vi "Autonomous Independent.vi"() -> ()   [LabVIEW 2017]
doc: "This VI is called when autonomous begins, and will automatically be terminated when autonomous ends. You can carry out timed or sensor driven robot movement independently without needing to return to the caller."
uses:
  <vilib>/Rock Robotics/Network Tables/NT Write Boolean.vi
  Robot Global Data.vi
  <vilib>/Rock Robotics/Network Tables/NT Read Number.vi
  <vilib>/Rock Robotics/WPI/Utilities/WPI_GetSetVariantRefNum.vi
  <vilib>/addons/control/pid/pid.llb/PID (DBL).vi
  <vilib>/Rock Robotics/WPI/RobotDrive/WPI_RobotDriveArcadeDrive_Standard(NoSaturation).vi
  <vilib>/Rock Robotics/Network Tables/NT Read Boolean.vi
  <vilib>/Rock Robotics/Network Tables/NT Write Number.vi
  <vilib>/addons/control/pid/NI_PID_pid.lvlib
panel:
  in  "PID turn angle gains":T1={"proportional gain (Kc)"=0.07, "integral time (Ti, min)"=0.0, "derivative time (Td, min)"=1e-05}
  in  "PID arm gains":T1={"proportional gain (Kc)"=1.1, "integral time (Ti, min)"=0.008, "derivative time (Td, min)"=0.0001}
  in  "PID control on":bool
  in  "Angle A?":bool=TRUE
  in  "angle A 2":dbl=30.0
  in  "angle B 2":dbl=90.0
  out "Waveform Chart arm":cluster{"angle B 2":dbl, "Arm Angle":dbl, dbl}(graph)
  in  "Chart slowing 2":i32(knob)=3 scale=1.0..10.0
  in  "Shooter control":dbl(slide) scale=-1.0..1.0
  in  "Arm control":dbl(slide) scale=-1.0..1.0
  in  "Chart slowing":i32(knob)=1 scale=1.0..10.0
  in  "angle B":dbl=90.0
  in  "angle A":dbl
  in  "Reset Gyro":bool
  out "Waveform Chart":cluster{"f":dbl, dbl}(graph)
  in  "Which angle?":bool=TRUE
  out "Stop Wheel Loop":bool
  # "Be sure to right-click and choose Data Operations>>Make Current Value default if you want to save the array values with the VI"
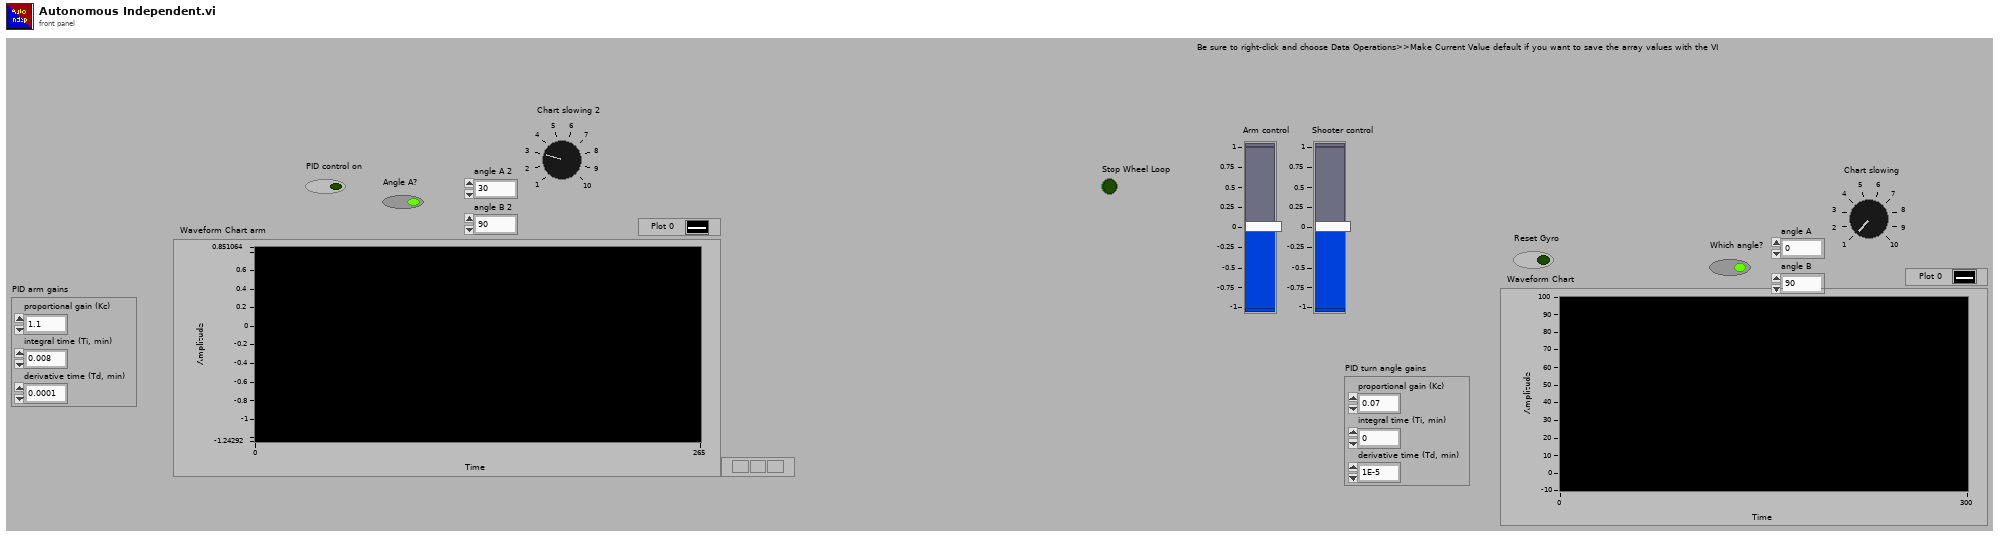
[diagram p1: front panel]
types:
  T1 = cluster{"proportional gain (Kc)":dbl, "integral time (Ti, min)":dbl, "derivative time (Td, min)":dbl}
  T2 = typedef "WPI_GyroDevRef.ctl" = cluster{"DevStatus":errorcluster, "Analog Channel":T3, "Gain (VoltsPerDegree/Second)":dbl, "Gyro Type":enum16{"Analog", "XRS450"}, "Handle":i32, "SPI Bus":T4, "Device Found":bool, "Sample Rate":dbl, "Calibrate On Open":bool, "Offset":dbl}
  T3 = typedef "FPGA_AIChannel.ctl" = enum8{"AI 0", "AI 1", "AI 2", "AI 3", "AI MXP 0", "AI MXP 1", "AI MXP 2", "AI MXP 3", "Invalid"}
  T4 = typedef "spi_bus.ctl" = enum16{"SPI On-Board, CS0", "SPI On-Board, CS1", "SPI On-Board, CS2", "SPI On-Board, CS3", "SPI MXP", "Invalid"}
  T5 = typedef "WPI_PotentiometerDevRef.ctl" = cluster{"DevStatus":errorcluster, "Analog Channel":T3, "Invert Output":bool}
  T6 = typedef "WPI_RobotDriveDevRef.ctl" = cluster{"DevStatus":errorcluster, "Motors[]":T7[], "Square Inputs":bool, "Max Output":dbl}
  T7 = typedef "WPI_MotorControlDeviceRef.ctl" = cluster{"DeviceStatus":errorcluster, "Type":T8, "PWM":cluster{"PWM Channel":T9, "DeadBand":T10}, "CAN":cluster{"Device Number":u8, "SetOutput VI Ref":variant, "GetOutput VI Ref":variant, "Enable VI Ref":variant, "Disable VI Ref":variant, "Data":variant}, "Invert":bool, "DIO PWM":cluster{"PWM \"Enable\" Channel":T9, "DIOChannel":T11, "PWM Rate":dbl}}
  T8 = typedef "WPI_MotorControlType.ctl" = enum16{"PWM", "CAN", "DIO PWM"}
  T9 = typedef "FPGA_DIOPWMChannel.ctl" = enum8{"PWM 0", "PWM 1", "PWM 2", "PWM 3", "PWM 4", "PWM 5", "PWM 6", "PWM 7", "PWM 8", "PWM 9", "PWM MXP 0", "PWM MXP 1", "PWM MXP 2", "PWM MXP 3", "PWM MXP 4", "PWM MXP 5", "PWM MXP 6", "PWM MXP 7", "PWM MXP 8", "PWM MXP 9", "Invalid"}
  T10 = typedef "WPI_PWMDeadband.ctl" = cluster{"Name":string, "maxPositivePwm":i32, "minPositivePwm":i32, "centerPwm":i32, "maxNegativePwm":i32, "minNegativePwm":i32, "angularRange":u16}
  T11 = typedef "FPGA_DIOChannel.ctl" = enum8{"DIO 0", "DIO 1", "DIO 2", "DIO 3", "DIO 4", "DIO 5", "DIO 6", "DIO 7", "DIO 8", "DIO 9", "DIO MXP 0", "DIO MXP 1", "DIO MXP 2", "DIO MXP 3", "DIO MXP 4", "DIO MXP 5", "DIO MXP 6", "DIO MXP 7", "DIO MXP 8", "DIO MXP 9", "DIO MXP 10", "DIO MXP 11", "DIO MXP 12", "DIO MXP 13", "DIO MXP 14", "DIO MXP 15", "SPI Port CS1", "SPI Port CS2", "SPI Port CS3", "SPI Port MISO", "SPI Port MOSI", "Invalid"}
  T12 = typedef "WPI_SwitchDevRef.ctl" = cluster{"DevStatus":errorcluster, "DIO Channel":T11, "CntIndex":T13, "Normally Closed":bool}
  T13 = typedef "FPGA_CounterCtrSystemIndex.ctl" = enum8{"Ctr 0", "Ctr 1", "Ctr 2", "Ctr 3", "Ctr 4", "Ctr 5", "Ctr 6", "Ctr 7", "Invalid"}
  T14 = typedef "WPI_AccelerometerDevRef.ctl" = cluster{"DevStatus":errorcluster, "Scaling":T15, "Analog Channels":T16, "I2C Bus":T17, "SPI Bus":T4, "Accel Range":T18, "ADXL Axes":T19, "Handle":i32, "Device Address":u8, "Accel Type":enum16{"Analog", "ADXL345 I2C", "ADXL345 SPI", "Internal", "ADXL362 SPI"}}
  T15 = typedef "WPI_AccelerometerScaling.ctl" = cluster{"Gain (VoltsPerG)":dbl, "Center Voltage":dbl}
  T16 = typedef "WPI_AccelerometerAnalogChannels.ctl" = cluster{"X-Axis":T3, "Y-Axis":T3, "Z-Axis":T3}
  T17 = typedef "i2c_bus.ctl" = enum16{"I2C On-Board", "I2C MXP", "Invalid"}
  T18 = typedef "ADXL345 Range.ctl" = u8
  T19 = typedef "WPI_AccelerometerADXL345 Axes.ctl" = cluster{"X-Axis":bool, "Y-Axis":bool, "Z-Axis":bool}
  T20 = cluster{"X-Axis":dbl, "Y-Axis":dbl, "Z-Axis":dbl}
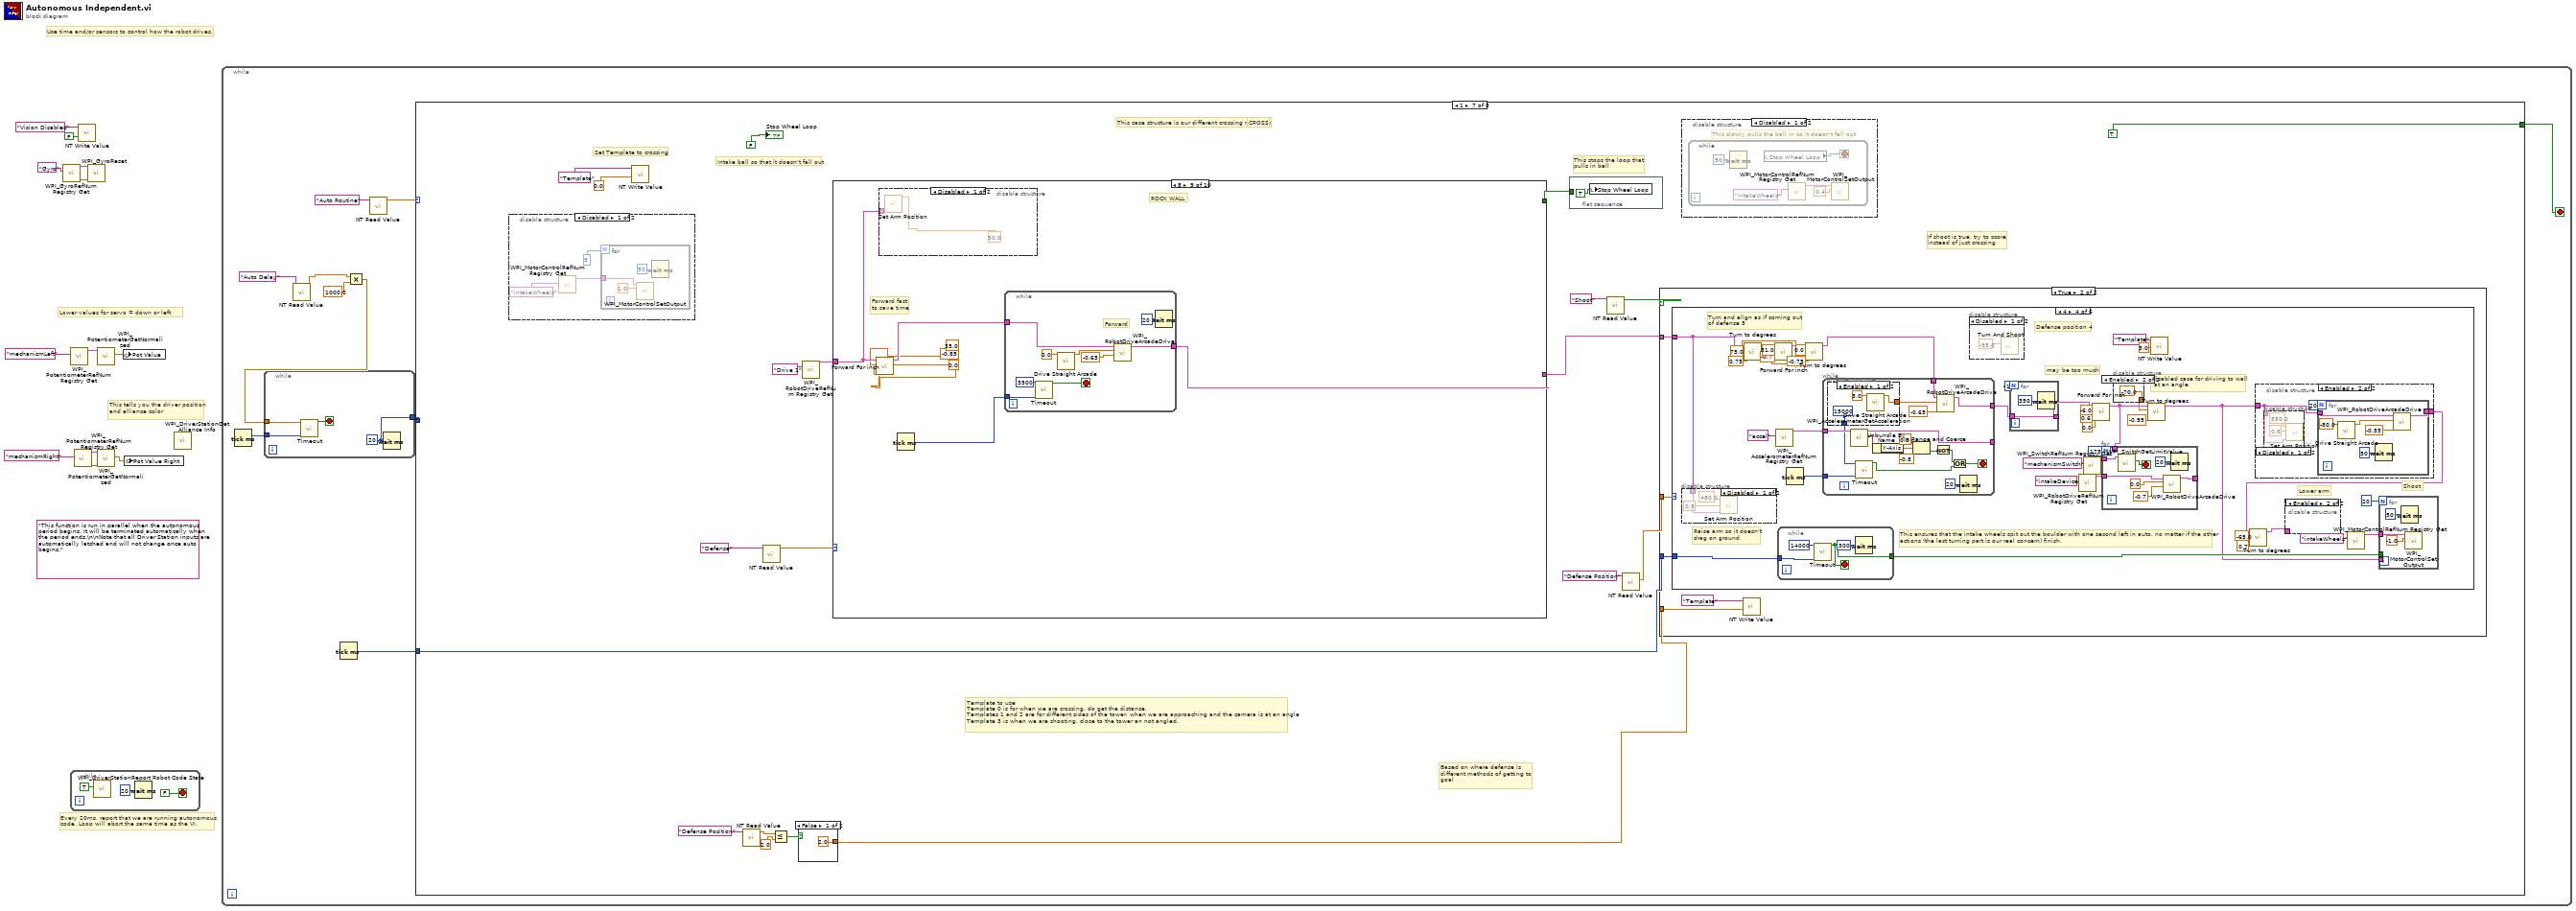
[diagram p0: block diagram]
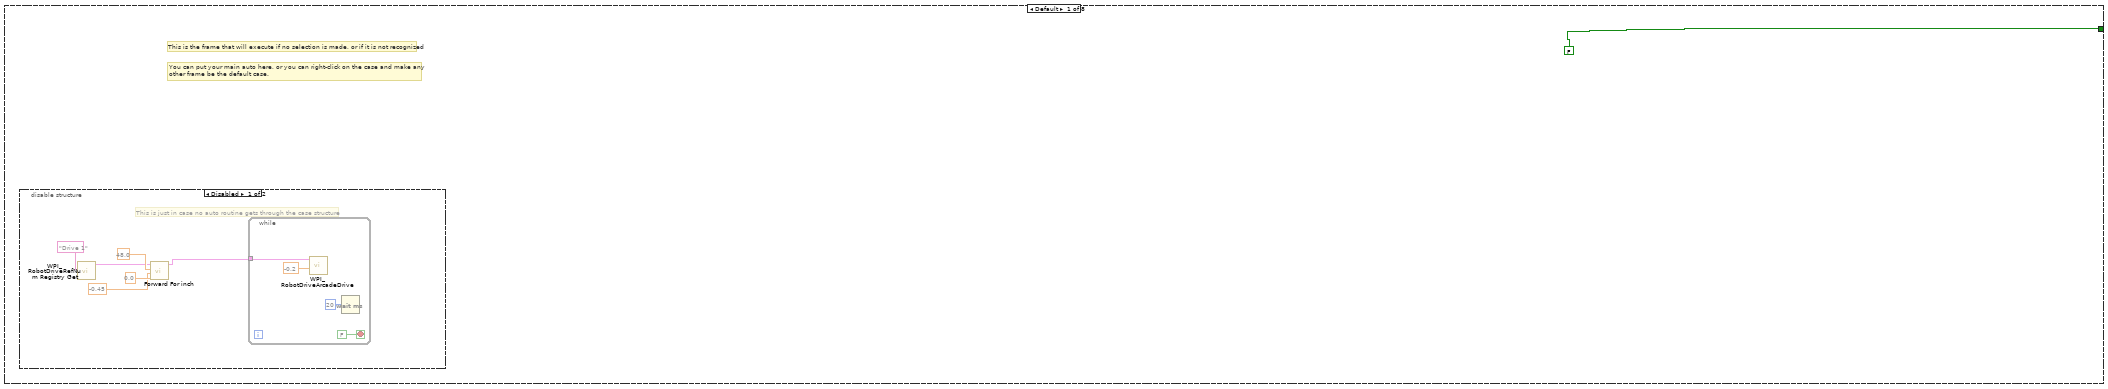
[diagram p2: hidden frame]
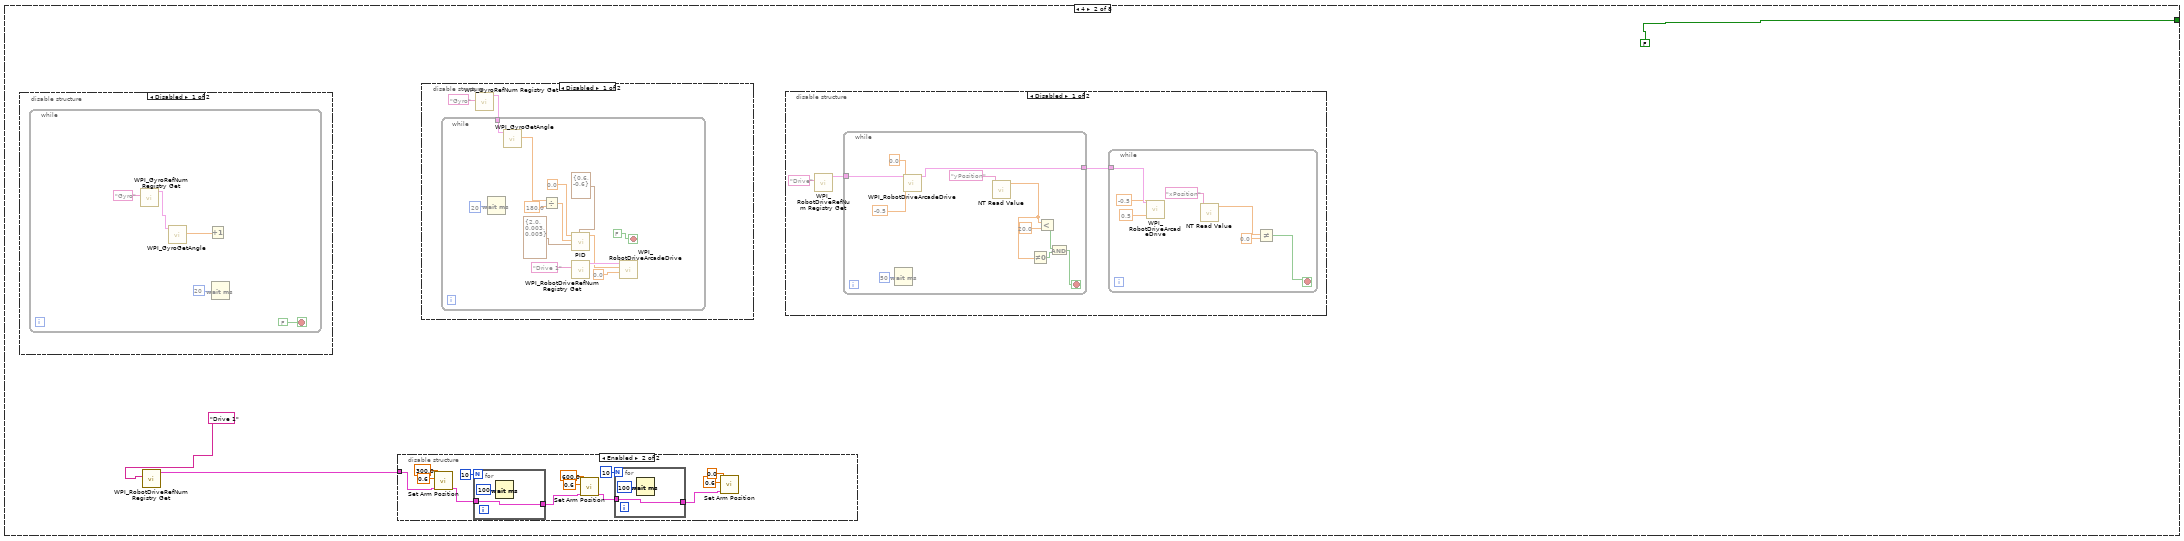
[diagram p4: hidden frame]
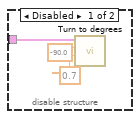
[diagram p5: hidden frame]
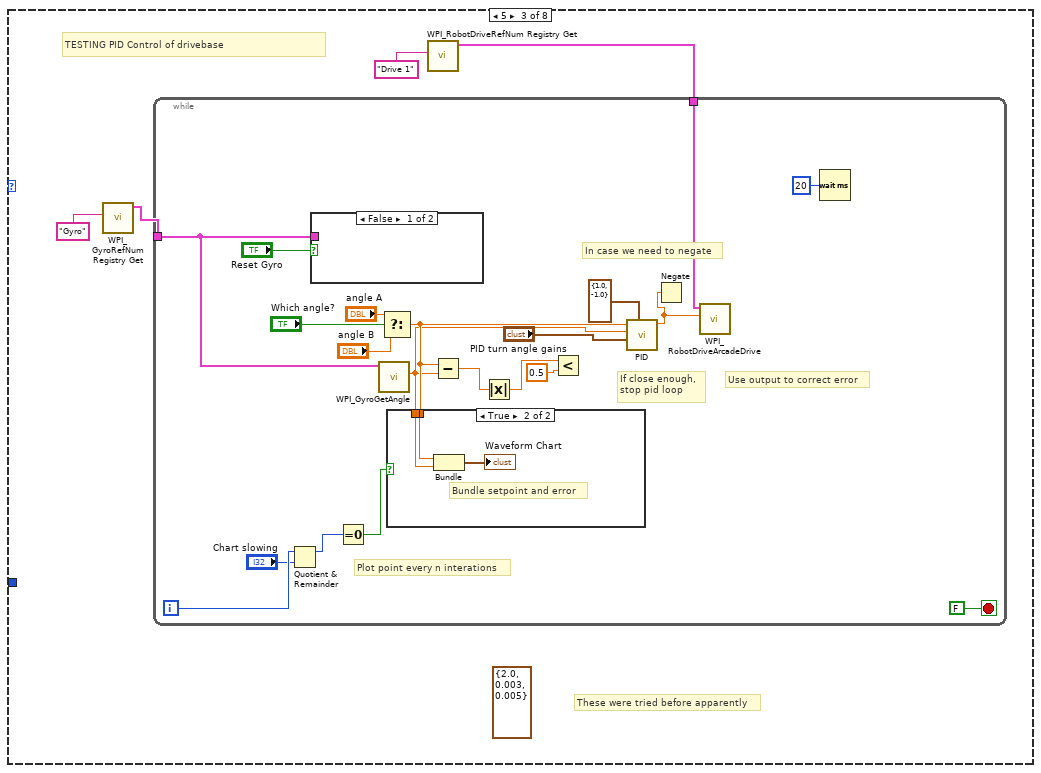
[diagram p9: hidden frame]
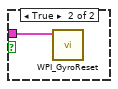
[diagram p11: hidden frame]
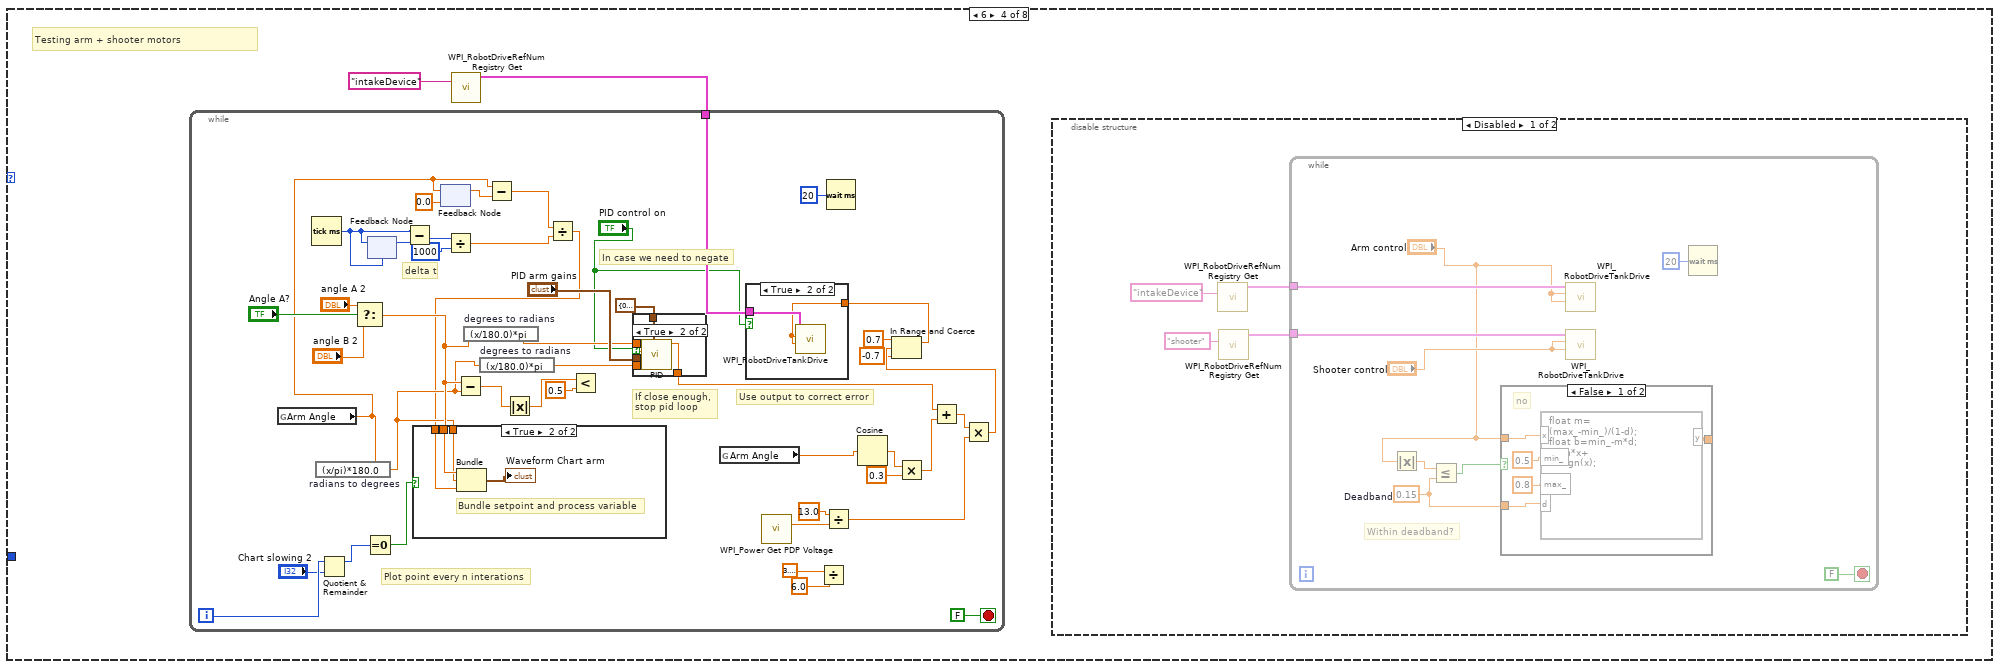
[diagram p12: hidden frame]
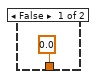
[diagram p14: hidden frame]
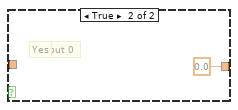
[diagram p16: hidden frame]
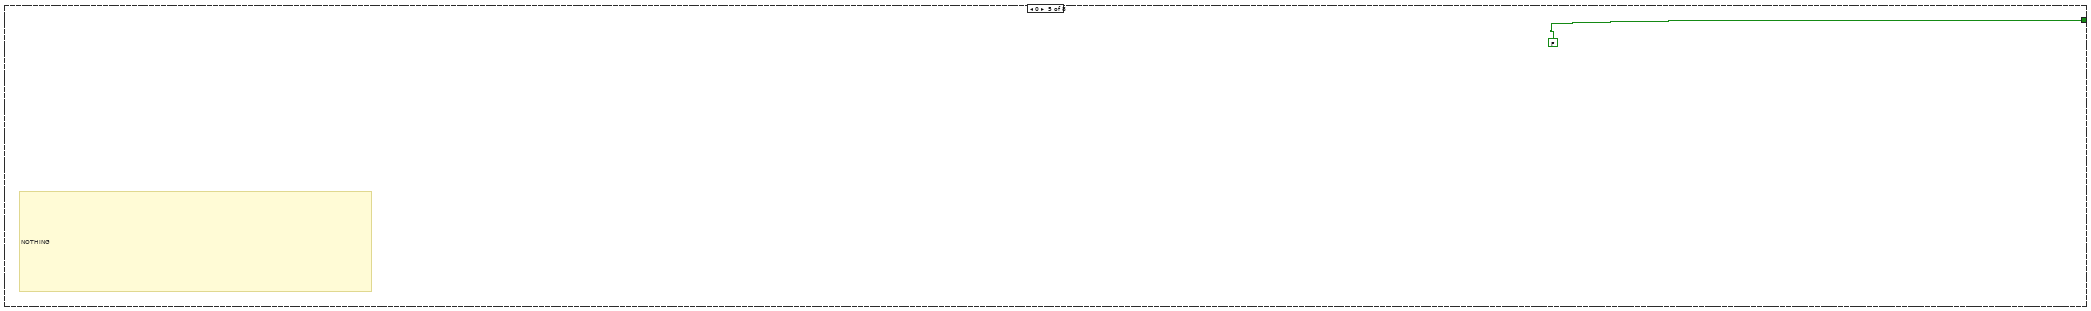
[diagram p18: hidden frame]
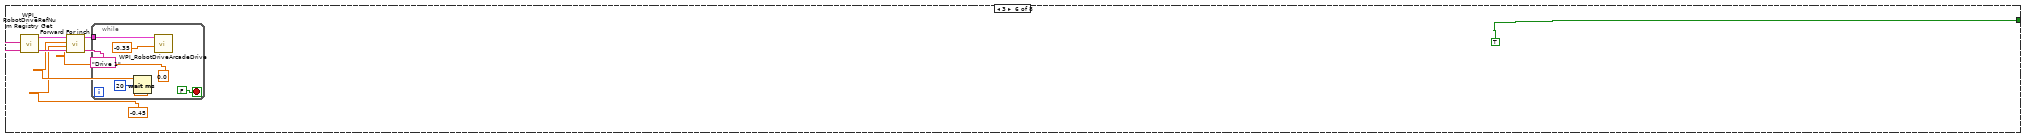
[diagram p19: hidden frame]
diagram:
  (unwired) "This function is run in parallel when the autonomous period begins. It will be terminated automatically when the period ends.\n\nNote that all Driver Station inputs are automatically latched and will not change once auto begins."
  # "Lower values for servo = down or left"
  # "Use time and/or sensors to control how the robot drives."
  # "Every 20ms, report that we are running autonomous\ncode. Loop will abort the same time as the VI."
  # "This tells you the driver position\nand alliance color"
  n1 = call <vilib>:"WPI_GyroRefNum Registry Get.vi"("refnum name"="Gyro") -> ("error out"=w12:errorcluster, "GyroDevRef"=w11:T2)  [unwired: 9 in]
  n2 = while {
    stop <- FALSE stop-if-true
    n3 = call <vilib>:"WPI_DriverStationReport Robot Code State.vi"("Autonomous"=TRUE) -> ()  [unwired: 10 in, 1 out]
    n4 = Wait (ms)(milliseconds to wait=u32 20) -> ()  [unwired: 1 out]
  }
  n5 = call <vilib>:"WPI_PotentiometerRefNum Registry Get.vi"("refnum name"="mechanismLeft") -> ("PotDevRef"=w4:T5)  [unwired: 9 in, 1 out]
  n6 = call <vilib>:"WPI_PotentiometerRefNum Registry Get.vi"("refnum name"="mechanismRight") -> ("error out"=w3:errorcluster, "PotDevRef"=w2:T5)  [unwired: 9 in]
  n7 = call-poly <vilib>:"NT Write Value.vi"("Boolean"=FALSE, "Name"="Vision Disabled") -> ()  [unwired: 9 in, 1 out]
  n8 = call <vilib>:"WPI_GyroReset.vi"("error in"=w12, "GyroDevRef"=w11) -> ()  [unwired: 8 in, 2 out]
  n9 = call <vilib>:"WPI_PotentiometerGetNormalized.vi"("PotDevRef"=w4) -> ("Normalized Value"=w7:dbl)  [unwired: 8 in, 2 out]
  n10 = call <vilib>:"WPI_PotentiometerGetNormalized.vi"("error in"=w3, "PotDevRef"=w2) -> ("Normalized Value"=w1:dbl)  [unwired: 7 in, 2 out]
  n11 = global write "Robot Global Data.vi" "Pot Value"(w7) -> ()
  n12 = global write "Robot Global Data.vi" "Pot Value Right"(w1) -> ()
  n13 = call <vilib>:"WPI_DriverStationGet Alliance Info.vi"() -> ()  [unwired: 12 out]
  n14 = while {
    stop <- w24 stop-if-true
    n15 = Tick Count (ms)() -> (millisecond timer value=w23:u32)
    n16 = call-poly <vilib>:"NT Read Value.vi"("Name"="Auto Delay") -> ("Numeric"=w20:dbl)  [unwired: 9 in, 1 out]
    n17 = Tick Count (ms)() -> (millisecond timer value=w17:u32)
    n18 = Multiply(x=w20, y=1000.0) -> (x*y=w18:dbl)
    n19 = while {
      tunnel: w23 -> [w29]
      tunnel: [w27] -> w22
      tunnel: w18 -> [w26]
      stop <- w28 stop-if-true
      w27 = u32 20 ("milliseconds to wait")
      n20 = call "Timeout.vi"("Start Time In"=w29, "Time Limit"=w26) -> ("Timeout"=w28:bool)  [unwired: 8 in, 1 out]
      n21 = Wait (ms)(milliseconds to wait=w27) -> ()  [unwired: 1 out]
    }
    n22 = call-poly <vilib>:"NT Read Value.vi"("Name"="Auto Routine") -> ("Numeric"=w16:dbl)  [unwired: 9 in, 1 out]
    n23 = case shown="1" w16 {
      tunnel: [FALSE FALSE _ _ FALSE TRUE TRUE TRUE] -> w24
      tunnel: w22 -> [_ _ _ _ _ _ _ _]
      tunnel: w17 -> [_ _ _ _ _ _ w223 _]
      frame Default {
        # "You can put your main auto here, or you can right-click on the case and make any\nother frame be the default case."
        # "This is the frame that will execute if no selection is made, or if it is not recognized"
        n24 = disable-structure shown="Disabled" {
          frame Disabled {
            # "This is just in case no auto routine gets through the case structure"
            n25 = call <vilib>:"WPI_RobotDriveRefNum Registry Get.vi"("refnum name"="Drive 1") -> ("RobotDriveDevRef"=w32:T6)  [unwired: 9 in, 1 out]
            n26 = call "Forward For inch.vi"("Angle robot facing"=0.0, "Speed"=-0.45, "Distance"=48.0, "RobotDriveDevRef in"=w32) -> ("RobotDriveDevRef out"=w36:T6)  [unwired: 7 in]
            n27 = while {
              tunnel: w36 -> [w38]
              stop <- FALSE stop-if-true
              n28 = call-poly <vilib>:"WPI_RobotDriveArcadeDrive.vi"("Y axis value"=-0.2, "RobotDriveDevRef"=w38) -> ()  [unwired: 7 in, 3 out]
              n29 = Wait (ms)(milliseconds to wait=u32 20) -> ()  [unwired: 1 out]
            }
          }
          frame Enabled {
          }
        }
      }
      frame 4 {
        n30 = disable-structure shown="Disabled" {
          frame Disabled {
            n31 = while {
              stop <- FALSE stop-if-true
              n32 = call <vilib>:"WPI_GyroRefNum Registry Get.vi"("refnum name"="Gyro") -> ("GyroDevRef"=w65:T2)  [unwired: 9 in, 1 out]
              n33 = call <vilib>:"WPI_GyroGetAngle.vi"("GyroDevRef"=w65) -> ("Angle"=w66:dbl)  [unwired: 6 in, 4 out]
              n34 = Increment(x=w66) -> ()  [unwired: 1 out]
              n35 = Wait (ms)(milliseconds to wait=u32 20) -> ()  [unwired: 1 out]
            }
          }
          frame Enabled {
          }
        }
        n36 = call <vilib>:"WPI_RobotDriveRefNum Registry Get.vi"("refnum name"="Drive 1") -> ("RobotDriveDevRef"=w41:T6)  [unwired: 9 in, 1 out]
        n37 = disable-structure shown="Enabled" {
          disable-tunnel: w41 -> [w44 w59]
          frame Disabled {
            n38 = call "Turn to degrees.vi"("Speed/Direction"=0.7, "Angle"=-90.0, "RobotDriveDevRef in"=w44) -> ()  [unwired: 8 in, 1 out]
          }
          frame Enabled {
            n39 = call "Set Arm Position.vi"("RobotDriveDevRef 2"=w59, "Speed"=0.6, "Setpoint"=300.0) -> ("RobotDriveDevRef"=w52:T6)  [unwired: 8 in]
            n40 = for {
              N: 10 -> [_]
              tunnel: [w62] -> w53
              tunnel: w52 -> [w62]
              n41 = Wait (ms)(milliseconds to wait=u32 100) -> ()  [unwired: 1 out]
            }
            n42 = call "Set Arm Position.vi"("RobotDriveDevRef 2"=w53, "Speed"=0.6, "Setpoint"=600.0) -> ("RobotDriveDevRef"=w47:T6)  [unwired: 8 in]
            n43 = for {
              N: 10 -> [_]
              tunnel: [w60] -> w48
              tunnel: w47 -> [w60]
              n44 = Wait (ms)(milliseconds to wait=u32 100) -> ()  [unwired: 1 out]
            }
            n45 = call "Set Arm Position.vi"("RobotDriveDevRef 2"=w48, "Speed"=0.6, "Setpoint"=0.0) -> ()  [unwired: 8 in, 1 out]
          }
        }
        n46 = disable-structure shown="Disabled" {
          frame Disabled {
            n47 = call <vilib>:"WPI_GyroRefNum Registry Get.vi"("refnum name"="Gyro") -> ("GyroDevRef"=w90:T2)  [unwired: 9 in, 1 out]
            n48 = while {
              tunnel: w90 -> [w101]
              stop <- FALSE stop-if-true
              n49 = Wait (ms)(milliseconds to wait=u32 20) -> ()  [unwired: 1 out]
              n50 = call <vilib>:"WPI_GyroGetAngle.vi"("GyroDevRef"=w101) -> ("Angle"=w103:dbl)  [unwired: 6 in, 4 out]
              n51 = Divide(x=w103, y=180.0) -> (x/y=w93:dbl)
              n52 = call-poly <vilib>:"PID.vi"("output range"=cluster{"output high":dbl, "output low":dbl} {"output high"=0.6, "output low"=-0.6}, "PID gains"=T1 {"proportional gain (Kc)"=2.0, "integral time (Ti, min)"=0.003, "derivative time (Td, min)"=0.005} ("Drive straight"), "process variable"=w93, "setpoint"=0.0) -> ("output"=w92:dbl)  [unwired: 6 in, 1 out]
              n53 = call <vilib>:"WPI_RobotDriveRefNum Registry Get.vi"("refnum name"="Drive 1") -> ("RobotDriveDevRef"=w99:T6)  [unwired: 1 in, 9 out]
              n54 = call-poly <vilib>:"WPI_RobotDriveArcadeDrive.vi"("Y axis value"=0.0, "X axis value"=w92, "RobotDriveDevRef"=w99) -> ()  [unwired: 6 in, 3 out]
            }
          }
          frame Enabled {
          }
        }
        n55 = disable-structure shown="Disabled" {
          frame Disabled {
            n56 = call <vilib>:"WPI_RobotDriveRefNum Registry Get.vi"("refnum name"="Drive") -> ("RobotDriveDevRef"=w70:T6)  [unwired: 9 in, 1 out]
            n57 = while {
              tunnel: w70 -> [w86]
              tunnel: [w84] -> w69
              stop <- w79 stop-if-true
              n58 = Wait (ms)(milliseconds to wait=u32 50) -> ()  [unwired: 1 out]
              n59 = call-poly <vilib>:"WPI_RobotDriveArcadeDrive.vi"("Y axis value"=-0.5, "X axis value"=0.0, "RobotDriveDevRef"=w86) -> ("RobotDriveDevRef"=w84:T6)  [unwired: 6 in, 2 out]
              n60 = call-poly <vilib>:"NT Read Value.vi"("Name"="yPosition") -> ("Numeric"=w81:dbl)  [unwired: 9 in, 1 out]
              n61 = Not Equal To 0?(x=w81) -> (x != 0?=w80:bool)
              n62 = Less?(x=w81, y=20.0) -> (x < y?=w82:bool)
              n63 = And(x=w82, y=w80) -> (x .and. y?=w79:bool)
            }
            n64 = while {
              tunnel: w69 -> [w78]
              stop <- w74 stop-if-true
              n65 = call-poly <vilib>:"WPI_RobotDriveArcadeDrive.vi"("Y axis value"=0.5, "X axis value"=-0.5, "RobotDriveDevRef"=w78) -> ()  [unwired: 6 in, 3 out]
              n66 = call-poly <vilib>:"NT Read Value.vi"("Name"="xPosition") -> ("Numeric"=w76:dbl)  [unwired: 9 in, 1 out]
              n67 = Not Equal?(x=w76, y=0.0) -> (x != y?=w74:bool)
            }
          }
          frame Enabled {
          }
        }
      }
      frame 5 {
        (unwired) T1 {"proportional gain (Kc)"=2.0, "integral time (Ti, min)"=0.003, "derivative time (Td, min)"=0.005} ("Drive straight")
        # "These were tried before apparently"
        # "TESTING PID Control of drivebase"
        n68 = call <vilib>:"WPI_GyroRefNum Registry Get.vi"("refnum name"="Gyro") -> ("GyroDevRef"=w108:T2)  [unwired: 9 in, 1 out]
        n69 = call <vilib>:"WPI_RobotDriveRefNum Registry Get.vi"("refnum name"="Drive 1") -> ("RobotDriveDevRef"=w105:T6)  [unwired: 9 in, 1 out]
        n70 = while {
          tunnel: w108 -> [w112]
          tunnel: w105 -> [w111]
          i -> [w114]
          stop <- FALSE stop-if-true
          # "In case we need to negate"
          # "Plot point every n interations"
          # "If close enough,\nstop pid loop"
          # "Use output to correct error"
          n71 = Quotient & Remainder(x=w114, y="Chart slowing") -> (x-y*floor(x/y)=w116:i32)  [unwired: 1 out]
          n72 = case shown="False" "Reset Gyro" {
            tunnel: w112 -> [_ w132]
            frame False {
            }
            frame True {
              n73 = call <vilib>:"WPI_GyroReset.vi"("GyroDevRef"=w132) -> ()  [unwired: 9 in, 2 out]
            }
          }
          n74 = Equal To 0?(x=w116) -> (x = 0?=w115:bool)
          n75 = call <vilib>:"WPI_GyroGetAngle.vi"("GyroDevRef"=w112) -> ("Angle"=w124:dbl)  [unwired: 6 in, 4 out]
          n76 = Select(t="angle A", s="Which angle?", f="angle B") -> (s? t:f=w126:dbl)
          n77 = case shown="True" w115 {
            tunnel: w126 -> [_ w130]
            tunnel: w124 -> [_ w129]
            frame False {
            }
            frame True {
              # "Bundle setpoint and error"
              n78 = Bundle("angle B"=w130, "Angle"=w129) -> (→"Waveform Chart":cluster{"angle B":dbl, "Angle":dbl})  [unwired: 1 in]
            }
          }
          n79 = Subtract(x=w126, y=w124) -> (x-y=w122:dbl)
          n80 = Absolute Value(x=w122) -> (abs(x)=w121:dbl)
          n81 = Less?(x=w121, y=0.5) -> ()  [unwired: 1 out]
          n82 = call-poly <vilib>:"PID.vi"("output range"=cluster{"output high":dbl, "output low":dbl} {"output high"=1.0, "output low"=-1.0}, "PID gains"="PID turn angle gains", "process variable"=w124, "setpoint"=w126) -> ("output"=w110:dbl)  [unwired: 6 in, 1 out]
          n83 = Negate(x=w110) -> ()  [unwired: 1 out]
          n84 = call-poly <vilib>:"WPI_RobotDriveArcadeDrive.vi"("X axis value"=w110, "RobotDriveDevRef"=w111) -> ()  [unwired: 7 in, 3 out]
          n85 = Wait (ms)(milliseconds to wait=u32 20) -> ()  [unwired: 1 out]
        }
      }
      frame 6 {
        # "Testing arm + shooter motors"
        n86 = call <vilib>:"WPI_RobotDriveRefNum Registry Get.vi"("refnum name"="intakeDevice") -> ("RobotDriveDevRef"=w134:T6)  [unwired: 9 in, 1 out]
        n87 = while {
          tunnel: w134 -> [w166]
          i -> [w168]
          stop <- FALSE stop-if-true
          # "delta t"
          # "In case we need to negate"
          # "Plot point every n interations"
          # "If close enough,\nstop pid loop"
          # "Use output to correct error"
          n88 = global read "Robot Global Data.vi" "Arm Angle"() -> (w136:dbl)
          n89 = Tick Count (ms)() -> (millisecond timer value=w143:u32)
          n90 = expression code="(x/pi)*180.0" "radians to degrees"(w136) -> (w145:dbl)
          n91 = Quotient & Remainder(x=w168, y="Chart slowing 2") -> (x-y*floor(x/y)=w170:i32)  [unwired: 1 out]
          n92 = Select(t="angle A 2", s="Angle A?", f="angle B 2") -> (s? t:f=w160:dbl)
          n93 = Equal To 0?(x=w170) -> (x = 0?=w169:bool)
          n94 = feedback #1(w143) -> (w144:u32)
          n95 = feedback-in #1(w143) -> ()
          n96 = Subtract(x=w143, y=w144) -> (x-y=w142:u32)
          n97 = feedback #2(0.0 ("Arm Angle")) -> (w140:dbl)
          n98 = feedback-in #2(w136) -> ()
          n99 = Divide(x=w142, y=u32 1000) -> (x/y=w137:dbl)
          n100 = Subtract(x=w160, y=w145) -> (x-y=w159:dbl)
          n101 = expression code="(x/180.0)*pi" "degrees to radians"(w160) -> (w161:dbl)
          n102 = expression code="(x/180.0)*pi" "degrees to radians"(w145) -> (w148:dbl)
          n103 = Subtract(x=w136, y=w140) -> (x-y=w138:dbl)
          n104 = Absolute Value(x=w159) -> (abs(x)=w175:dbl)
          n105 = Divide(x=w138, y=w137) -> (x/y=w135:dbl)
          n106 = case shown="True" w169 {
            tunnel: w160 -> [_ w191]
            tunnel: w145 -> [_ w190]
            tunnel: w135 -> [_ w188]
            frame False {
            }
            frame True {
              # "Bundle setpoint and process variable"
              n107 = Bundle("angle B 2"=w191, "Arm Angle"=w190, w188) -> (→"Waveform Chart arm":cluster{"angle B 2":dbl, "Arm Angle":dbl, dbl})  [unwired: 1 in]
            }
          }
          n108 = Less?(x=w175, y=0.5) -> ()  [unwired: 1 out]
          n109 = case shown="True" "PID control on" {
            tunnel: "PID arm gains" -> [_ w187]
            tunnel: cluster{"output high":dbl, "output low":dbl} {"output high"=0.7, "output low"=-0.7} ("output range") -> [_ w186]
            tunnel: w161 -> [_ w185]
            tunnel: w148 -> [_ w184]
            tunnel: [0.0 ("output") w183] -> w147
            frame False {
            }
            frame True {
              n110 = call-poly <vilib>:"PID.vi"("output range"=w186, "PID gains"=w187, "process variable"=w184, "setpoint"=w185) -> ("output"=w183:dbl)  [unwired: 6 in, 1 out]
            }
          }
          n111 = global read "Robot Global Data.vi" "Arm Angle"() -> (w155:dbl)
          n112 = call <vilib>:"WPI_Power Get PDP Voltage.vi"() -> ("voltage (V)"=w165:dbl)  [unwired: 14 in, 1 out]
          n113 = Divide(x=3.141592653589793, y=6.0) -> ()  [unwired: 1 out]
          n114 = Divide(x=13.0, y=w165) -> (x/y=w153:dbl)
          n115 = Wait (ms)(milliseconds to wait=u32 20) -> ()  [unwired: 1 out]
          n116 = Cosine(x=w155) -> (cos(x)=w158:dbl)
          n117 = Multiply(x=w158, y=0.3) -> (x*y=w156:dbl)
          n118 = Add(x=w147, y=w156) -> (x+y=w154:dbl)
          n119 = Multiply(x=w154, y=w153) -> (x*y=w152:dbl)
          n120 = In Range and Coerce(upper limit=0.7, x=w152, lower limit=-0.7) -> (coerced(x)=w149:dbl)  [unwired: 1 out]
          n121 = case shown="True" "PID control on" {
            tunnel: w166 -> [_ w181]
            tunnel: w149 -> [_ w180]
            frame False {
            }
            frame True {
              n122 = call <vilib>:"WPI_RobotDriveTankDrive.vi"("Right axis value"=w180, "Left axis value"=w180, "RobotDriveDevRef"=w181) -> ()  [unwired: 6 in, 3 out]
            }
          }
        }
        n123 = disable-structure shown="Disabled" {
          frame Disabled {
            n124 = call <vilib>:"WPI_RobotDriveRefNum Registry Get.vi"("refnum name"="intakeDevice") -> ("RobotDriveDevRef"=w195:T6)  [unwired: 9 in, 1 out]
            n125 = call <vilib>:"WPI_RobotDriveRefNum Registry Get.vi"("refnum name"="shooter") -> ("RobotDriveDevRef"=w194:T6)  [unwired: 9 in, 1 out]
            n126 = while {
              tunnel: w195 -> [w203]
              tunnel: w194 -> [w202]
              stop <- FALSE stop-if-true
              w198 = 0.15  # Deadband
              # "Within deadband?"
              n127 = Absolute Value(x="Arm control") -> (abs(x)=w200:dbl)
              n128 = Less Or Equal?(x=w200, y=w198) -> (x <= y?=w199:bool)
              n129 = case shown="False" w199 {
                tunnel: [w209 0.0 ("y")] -> _
                tunnel: "Arm control" -> [w206 _]
                tunnel: w198 -> [w205 _]
                frame False {
                  # "no"
                  n130 = formula code="float m= \n(max_-min_)/(1-d);\nfloat b=min_-m*d;\ny=m*x+\nb*sign(x);"("x"=w206, "min_"=0.5 ("input variable"), "max_"=0.8 ("input variable"), "d"=w205) -> ("y"=w209:dbl)
                }
                frame True {
                  # "Yes"
                  # "Output 0"
                }
              }
              n131 = call <vilib>:"WPI_RobotDriveTankDrive.vi"("Right axis value"="Arm control", "Left axis value"="Arm control", "RobotDriveDevRef"=w203) -> ()  [unwired: 6 in, 3 out]
              n132 = call <vilib>:"WPI_RobotDriveTankDrive.vi"("Right axis value"="Shooter control", "Left axis value"="Shooter control", "RobotDriveDevRef"=w202) -> ()  [unwired: 6 in, 3 out]
              n133 = Wait (ms)(milliseconds to wait=u32 20) -> ()  [unwired: 1 out]
            }
          }
          frame Enabled {
          }
        }
      }
      frame 0 {
        # "NOTHING"
      }
      frame 3 {
        n134 = call <vilib>:"WPI_RobotDriveRefNum Registry Get.vi"("refnum name"="Drive 1") -> ("RobotDriveDevRef"=w217:T6)  [unwired: 9 in, 1 out]
        n135 = call "Forward For inch.vi"("Angle robot facing"=0.0, "Speed"=-0.45, "Distance"=48.0, "RobotDriveDevRef in"=w217) -> ("RobotDriveDevRef out"=w213:T6)  [unwired: 7 in]
        n136 = while {
          tunnel: w213 -> [w220]
          stop <- FALSE stop-if-true
          n137 = Wait (ms)(milliseconds to wait=u32 20) -> ()  [unwired: 1 out]
          n138 = call-poly <vilib>:"WPI_RobotDriveArcadeDrive.vi"("Y axis value"=-0.35, "RobotDriveDevRef"=w220) -> ()  [unwired: 7 in, 3 out]
        }
      }
      frame 1 {
        # "CROSS"
        # "This stops the loop that\npulls in ball"
        # "Based on where defense is\ndifferent methods of getting to\ngoal"
        # "If shoot is true, try to score\ninstead of just crossing"
        # "This case structure is our different crossing methods"
        # "Intake ball so that it doesn't fall out"
        # "Set Template to crossing"
        # "Template to use\nTemplate 0 is for when we are crossing, do get the distance.\nTemplates 1 and 2 are for different sides of the tower, when we are approaching and the camera is at an angle\nTemplate 3 is when we are shooting, close to the tower an not angled."
        n139 = disable-structure shown="Disabled" {
          frame Disabled {
            n140 = call <vilib>:"WPI_MotorControlRefNum Registry Get.vi"("refnum name"="intakeWheels") -> ("MotorControlDevRef"=w248:T7)  [unwired: 9 in, 1 out]
            n141 = for {
              N: 5 -> [_]
              tunnel: w248 -> [w251]
              n142 = call <vilib>:"WPI_MotorControlSetOutput.vi"("Output"=1.0, "MotorControlDevRef"=w251) -> ()  [unwired: 7 in, 3 out]
              n143 = Wait (ms)(milliseconds to wait=u32 50) -> ()  [unwired: 1 out]
            }
          }
          frame Enabled {
          }
        }
        n144 = call-poly <vilib>:"NT Write Value.vi"("Numeric"=0.0, "Name"="Template") -> ()  [unwired: 9 in, 1 out]
        n145 = call-poly <vilib>:"NT Read Value.vi"("Name"="Defense Position") -> ("Numeric"=w229:dbl)  [unwired: 9 in, 1 out]
        n146 = call-poly <vilib>:"NT Read Value.vi"("Name"="Defense") -> ("Numeric"=w240:dbl)  [unwired: 9 in, 1 out]
        n147 = Less Or Equal?(x=w229, y=2.0) -> (x <= y?=w231:bool)
        n148 = case shown="False" w231 {
          tunnel: [2.0 ("Speed/Direction") 1.0 ("Speed/Direction")] -> w227
          frame False {
          }
          frame True {
          }
        }
        n149 = call <vilib>:"WPI_RobotDriveRefNum Registry Get.vi"("refnum name"="Drive 1") -> ("RobotDriveDevRef"=w238:T6)  [unwired: 9 in, 1 out]
        n150 = case shown="8" w240 {
          tunnel: [w257 w264 w290 w413 w500 w514 w528 w537 w554 w566] -> w232
          tunnel: w238 -> [w257 w269 w289 w414 w496 w513 w527 w538 w553 w568]
          tunnel: [FALSE _ _ _ _ _ _ _ _ _] -> w234
          frame 0, Default {
          }
          frame 1 {
            # "If we decide to drive to castle wall at an angle,\nthe code in the enabled structure will be disabled\nand code will be enabled in the next case structure\nit drive at an angle"
            # "Lower arm"
            # "Go under bar, up to align with low goal"
            # "Go forward fast (to save time)"
            # "Pause"
            # "LOW BAR"
            n151 = call <vilib>:"WPI_SwitchRefNum Registry Get.vi"("refnum name"="mechanismSwitch") -> ("SwitchDevRef"=w260:T12)  [unwired: 9 in, 1 out]
            n152 = call <vilib>:"WPI_RobotDriveRefNum Registry Get.vi"("refnum name"="intakeDevice") -> ("RobotDriveDevRef"=w259:T6)  [unwired: 9 in, 1 out]
            n153 = for {
              N: 1 -> [_]
              tunnel: [w287] -> w265
              tunnel: w269 -> [w287]
              n154 = Wait (ms)(milliseconds to wait=u32 350) -> ()  [unwired: 1 out]
            }
            n155 = disable-structure shown="Enabled" {
              disable-tunnel: w269 -> [w279 _]
              disable-tunnel: w260 -> [_ w281]
              disable-tunnel: w259 -> [_ w280]
              frame Disabled {
                n156 = call "Set Arm Position.vi"("RobotDriveDevRef 2"=w279, "Speed"=0.95, "Setpoint"=510.0) -> ()  [unwired: 8 in, 1 out]
              }
              frame Enabled {
                n157 = while {
                  tunnel: w281 -> [w283]
                  tunnel: w280 -> [w282]
                  stop <- w284 stop-if-true
                  n158 = call <vilib>:"WPI_SwitchGetLimitValue.vi"("SwitchDevRef"=w283) -> ("Switch Pressed"=w284:bool)  [unwired: 8 in, 2 out]
                  n159 = call-poly <vilib>:"WPI_RobotDriveArcadeDrive.vi"("Y axis value"=-0.7, "X axis value"=0.0, "RobotDriveDevRef"=w282) -> ()  [unwired: 6 in, 3 out]
                }
              }
            }
            n160 = call "Forward For inch.vi"("Angle robot facing"=0.0, "Speed"=0.78, "Distance"=-32.0, "RobotDriveDevRef in"=w265) -> ("RobotDriveDevRef out"=w263:T6)  [unwired: 7 in]
            n161 = disable-structure shown="Enabled" {
              disable-tunnel: [w272 w276] -> w264
              disable-tunnel: w263 -> [w271 w276]
              frame Enabled {
                n162 = call "Forward For inch.vi"("Angle robot facing"=5.0, "Speed"=0.67, "Distance"=-172.0, "RobotDriveDevRef in"=w271) -> ("RobotDriveDevRef out"=w272:T6)  [unwired: 7 in]
              }
              frame Disabled {
              }
            }
          }
          frame 2 {
            # "PORTCULLIS"
            n163 = disable-structure shown="Enabled" {
              disable-tunnel: [w301 w363] -> w290
              disable-tunnel: w289 -> [w293 w378]
              frame Disabled {
                # "then pause while arm\nlowering"
                # "Pause"
                # "Because we had trouble making it go far\nenough, add a burst of movement at the end"
                # "We think the arm wasn't rasing\nbecause forward for inch wasn't\nending, so we added a time value instead"
                # "I'M SORRY THS IS SO COMPLICATED"
                # "Go forward slowly, so we \ndon't roll off ramp. When arm is high \nenough, start moving forward"
                # "raise arm, and porticullis"
                # "pause"
                # "Go forward to\nporticullus"
                # "Lower arm"
                n164 = for {
                  N: 1 -> [_]
                  tunnel: w293 -> [w358]
                  tunnel: [w358] -> w305
                  n165 = Wait (ms)(milliseconds to wait=u32 750) -> ()  [unwired: 1 out]
                }
                n166 = call "Set Arm Position.vi"("RobotDriveDevRef 2"=w293, "Speed"=0.7, "Setpoint"=700.0) -> ()  [unwired: 8 in, 1 out]
                n167 = global read "Robot Global Data.vi" "Pot Value"() -> (w297:dbl)
                n168 = call <vilib>:"WPI_PotentiometerRefNum Registry Get.vi"("refnum name"="mechanismLeft") -> ("PotDevRef"=w298:T5)  [unwired: 9 in, 1 out]
                n169 = call "Forward For inch.vi"("Angle robot facing"=0.0, "Speed"=-0.5, "Distance"=47.0, "RobotDriveDevRef in"=w305) -> ("RobotDriveDevRef out"=w308:T6)  [unwired: 7 in]
                n170 = call <vilib>:"WPI_RobotDriveRefNum Registry Get.vi"("refnum name"="Drive 1") -> ("RobotDriveDevRef"=w302:T6)  [unwired: 9 in, 1 out]
                n171 = flat-sequence {
                  tunnel: [w313] -> w300
                  tunnel: w294 -> [_]
                  frame #0 {
                    n172 = Tick Count (ms)() -> (millisecond timer value=w313:u32)
                  }
                }
                n173 = for {
                  N: 1 -> [_]
                  tunnel: w308 -> [w360]
                  tunnel: [w360] -> w294
                  n174 = Wait (ms)(milliseconds to wait=u32 200) -> ()  [unwired: 1 out]
                }
                n175 = while {
                  tunnel: w300 -> [w341]
                  tunnel: w294 -> [w336]
                  tunnel: [w335] -> w295
                  stop <- w339 stop-if-true
                  n176 = call "Timeout.vi"("Start Time In"=w341, "Time Limit"=u32 250) -> ("Timeout"=w339:bool)  [unwired: 8 in, 1 out]
                  n177 = call-poly <vilib>:"WPI_RobotDriveArcadeDrive.vi"("Y axis value"=-0.6, "X axis value"=0.0, "RobotDriveDevRef"=w336) -> ("RobotDriveDevRef"=w335:T6)  [unwired: 6 in, 2 out]
                }
                n178 = while {
                  tunnel: w295 -> [w348]
                  tunnel: [w348] -> w296
                  tunnel: w302 -> [w346]
                  tunnel: w298 -> [w345]
                  tunnel: w297 -> [w342]
                  stop <- w349 stop-if-true
                  n179 = call <vilib>:"WPI_PotentiometerGetNormalized.vi"("PotDevRef"=w345) -> ("Normalized Value"=w344:dbl)  [unwired: 8 in, 2 out]
                  n180 = disable-structure shown="Enabled" {
                    disable-tunnel: w344 -> [w352 w355]
                    disable-tunnel: [w351 w353] -> w343
                    disable-tunnel: w342 -> [_ w354]
                    frame Disabled {
                      n181 = expression code="-1505.88*(x-.587)"(w352) -> (w351:dbl)
                    }
                    frame Enabled {
                      n182 = Subtract(x=w355, y=w354) -> (x-y=w357:dbl)
                      n183 = Multiply(x=w357, y=-1505.88) -> (x*y=w353:dbl)
                    }
                  }
                  n184 = Less Or Equal?(x=w343, y=300.0) -> (x <= y?=w349:bool)
                  n185 = call-poly <vilib>:"WPI_RobotDriveArcadeDrive.vi"("Y axis value"=-0.45, "RobotDriveDevRef"=w346) -> ()  [unwired: 7 in, 3 out]
                }
                n186 = call "Set Arm Position.vi"("RobotDriveDevRef 2"=w295, "Speed"=0.8, "Setpoint"=150.0) -> ()  [unwired: 8 in, 1 out]
                n187 = disable-structure shown="Enabled" {
                  disable-tunnel: [w315 w327] -> w301
                  disable-tunnel: w296 -> [w314 w328]
                  frame Disabled {
                    # "Go forward"
                    n188 = Tick Count (ms)() -> (millisecond timer value=w319:u32)
                    n189 = while {
                      tunnel: w319 -> [w326]
                      tunnel: [24.0 ("Distance")] -> w316
                      stop <- w324 stop-if-true
                      n190 = call "Timeout.vi"("Start Time In"=w326, "Time Limit"=u32 10000) -> ("Timeout"=w324:bool)  [unwired: 8 in, 1 out]
                    }
                    n191 = call "Forward For inch.vi"("Angle robot facing"=0.0, "Speed"=-0.7, "Distance"=60.0, "RobotDriveDevRef in"=w314) -> ("RobotDriveDevRef out"=w315:T6)  [unwired: 7 in]
                    n192 = call "Forward For inch.vi"("Angle robot facing"=0.0, "Speed"=-0.65, "Distance"=w316, "RobotDriveDevRef in"=w315) -> ()  [unwired: 7 in, 1 out]
                  }
                  frame Enabled {
                    n193 = for {
                      N: 150 -> [_]
                      tunnel: w328 -> [w332]
                      tunnel: [w330] -> w327
                      n194 = call-poly <vilib>:"WPI_RobotDriveArcadeDrive.vi"("Y axis value"=-0.7, "X axis value"=0.0, "RobotDriveDevRef"=w332) -> ("RobotDriveDevRef"=w330:T6)  [unwired: 6 in, 2 out]
                      n195 = Wait (ms)(milliseconds to wait=u32 20) -> ()  [unwired: 1 out]
                    }
                  }
                }
              }
              frame Enabled {
                # "Go forward"
                # "Wait"
                # "Raise arm"
                # "Forward"
                # "Pause"
                # "Forward"
                # "Lower arm"
                # "Pause"
                n196 = for {
                  N: 1 -> [_]
                  tunnel: w378 -> [w405]
                  tunnel: [w405] -> w374
                  n197 = Wait (ms)(milliseconds to wait=u32 750) -> ()  [unwired: 1 out]
                }
                n198 = call <vilib>:"WPI_SwitchRefNum Registry Get.vi"("refnum name"="mechanismSwitch") -> ("SwitchDevRef"=w382:T12)  [unwired: 9 in, 1 out]
                n199 = call <vilib>:"WPI_RobotDriveRefNum Registry Get.vi"("refnum name"="intakeDevice") -> ("RobotDriveDevRef"=w381:T6)  [unwired: 9 in, 1 out]
                n200 = for {
                  N: 60 -> [_]
                  tunnel: w382 -> [w410]
                  tunnel: w381 -> [w409]
                  tunnel: w378 -> [_]
                  stop <- w408 stop-if-true
                  n201 = call <vilib>:"WPI_SwitchGetLimitValue.vi"("SwitchDevRef"=w410) -> ("Switch Pressed"=w408:bool)  [unwired: 8 in, 2 out]
                  n202 = call-poly <vilib>:"WPI_RobotDriveArcadeDrive.vi"("Y axis value"=-0.7, "X axis value"=0.0, "RobotDriveDevRef"=w409) -> ()  [unwired: 6 in, 3 out]
                  n203 = Wait (ms)(milliseconds to wait=u32 50) -> ()  [unwired: 1 out]
                }
                n204 = call "Forward For inch.vi"("Angle robot facing"=0.0, "Speed"=-0.6, "Distance"=46.0, "RobotDriveDevRef in"=w374) -> ("RobotDriveDevRef out"=w372:T6)  [unwired: 7 in]
                n205 = for {
                  N: 1 -> [_]
                  tunnel: w372 -> [w403]
                  tunnel: [w403] -> w371
                  n206 = Wait (ms)(milliseconds to wait=u32 200) -> ()  [unwired: 1 out]
                }
                n207 = for {
                  N: 6 -> [_]
                  tunnel: w371 -> [w387]
                  tunnel: [w386] -> w366
                  n208 = Wait (ms)(milliseconds to wait=u32 50) -> ()  [unwired: 1 out]
                  n209 = call-poly <vilib>:"WPI_RobotDriveArcadeDrive.vi"("Y axis value"=-0.6, "X axis value"=0.0, "RobotDriveDevRef"=w387) -> ("RobotDriveDevRef"=w386:T6)  [unwired: 6 in, 2 out]
                }
                n210 = call <vilib>:"WPI_RobotDriveRefNum Registry Get.vi"("refnum name"="intakeDevice") -> ("RobotDriveDevRef"=w368:T6)  [unwired: 9 in, 1 out]
                n211 = for {
                  N: 50 -> [_]
                  tunnel: w366 -> [_]
                  tunnel: w368 -> [w399]
                  n212 = call-poly <vilib>:"WPI_RobotDriveArcadeDrive.vi"("Y axis value"=0.8, "X axis value"=0.0, "RobotDriveDevRef"=w399) -> ()  [unwired: 6 in, 3 out]
                  n213 = Wait (ms)(milliseconds to wait=u32 50) -> ()  [unwired: 1 out]
                }
                n214 = for {
                  N: 40 -> [_]
                  tunnel: w366 -> [w395]
                  tunnel: [w395] -> w364
                  n215 = Wait (ms)(milliseconds to wait=u32 20) -> ()  [unwired: 1 out]
                  n216 = call-poly <vilib>:"WPI_RobotDriveArcadeDrive.vi"("Y axis value"=-0.55, "X axis value"=0.0, "RobotDriveDevRef"=w395) -> ()  [unwired: 6 in, 3 out]
                }
                n217 = for {
                  N: 90 -> [_]
                  tunnel: w364 -> [w392]
                  tunnel: [w390] -> w363
                  n218 = call-poly <vilib>:"WPI_RobotDriveArcadeDrive.vi"("Y axis value"=-0.85, "X axis value"=0.0, "RobotDriveDevRef"=w392) -> ("RobotDriveDevRef"=w390:T6)  [unwired: 6 in, 2 out]
                  n219 = Wait (ms)(milliseconds to wait=u32 20) -> ()  [unwired: 1 out]
                }
              }
            }
          }
          frame 3 {
            # "CDF"
            n220 = disable-structure shown="Enabled" {
              disable-tunnel: w414 -> [w429 w459]
              disable-tunnel: [w415 w445] -> w413
              frame Disabled {
                # "Raise arm so it doesn't hit the ground"
                # "Go over"
                # "Very small pause"
                # "While going forward so\nwe don't roll off"
                # "Lower arm onto CDF"
                # "Forward"
                n221 = call "Forward For inch.vi"("Angle robot facing"=0.0, "Speed"=-0.6, "Distance"=38.5, "RobotDriveDevRef in"=w429) -> ("RobotDriveDevRef out"=w420:T6)  [unwired: 7 in]
                n222 = call "Set Arm Position.vi"("RobotDriveDevRef 2"=w420, "Speed"=0.9, "Setpoint"=650.0) -> ("RobotDriveDevRef"=w419:T6)  [unwired: 8 in]
                n223 = for {
                  N: 50 -> [_]
                  tunnel: w420 -> [w432]
                  n224 = Wait (ms)(milliseconds to wait=u32 20) -> ()  [unwired: 1 out]
                  n225 = call-poly <vilib>:"WPI_RobotDriveArcadeDrive.vi"("Y axis value"=-0.35, "X axis value"=0.0 ("Y axis value"), "RobotDriveDevRef"=w432) -> ()  [unwired: 6 in, 3 out]
                }
                n226 = Tick Count (ms)() -> (millisecond timer value=w416:u32)
                n227 = for {
                  N: 5 -> [_]
                  tunnel: [w430] -> w421
                  tunnel: w419 -> [w430]
                  n228 = Wait (ms)(milliseconds to wait=u32 50) -> ()  [unwired: 1 out]
                }
                n229 = while {
                  tunnel: w419 -> [w443]
                  tunnel: [w442] -> w415
                  tunnel: w416 -> [w439]
                  stop <- w438 stop-if-true
                  n230 = call "Timeout.vi"("Start Time In"=w439, "Time Limit"=u32 4000) -> ("Timeout"=w438:bool)  [unwired: 8 in, 1 out]
                  n231 = call "Drive Straight Arcade.vi"("Angle robot facing"=0.0) -> ("Arcade drive x"=w436:dbl)  [unwired: 10 in]
                  n232 = call-poly <vilib>:"WPI_RobotDriveArcadeDrive.vi"("Y axis value"=-0.65, "X axis value"=w436, "RobotDriveDevRef"=w443) -> ("RobotDriveDevRef"=w442:T6)  [unwired: 6 in, 2 out]
                  n233 = Wait (ms)(milliseconds to wait=u32 20) -> ()  [unwired: 1 out]
                }
                n234 = call "Set Arm Position.vi"("RobotDriveDevRef 2"=w421, "Speed"=0.9, "Setpoint"=200.0) -> ()  [unwired: 8 in, 1 out]
              }
              frame Enabled {
                # "forward"
                # "arm up"
                # "While going forward so\nwe don't roll off"
                n235 = call "Forward For inch.vi"("Angle robot facing"=0.0, "Speed"=-0.6, "Distance"=38.0, "RobotDriveDevRef in"=w459) -> ("RobotDriveDevRef out"=w455:T6)  [unwired: 7 in]
                n236 = call <vilib>:"WPI_SwitchRefNum Registry Get.vi"("refnum name"="mechanismSwitch") -> ("SwitchDevRef"=w452:T12)  [unwired: 9 in, 1 out]
                n237 = for {
                  N: 50 -> [_]
                  tunnel: w455 -> [w487]
                  n238 = Wait (ms)(milliseconds to wait=u32 20) -> ()  [unwired: 1 out]
                  n239 = call-poly <vilib>:"WPI_RobotDriveArcadeDrive.vi"("Y axis value"=-0.35, "X axis value"=0.0 ("Y axis value"), "RobotDriveDevRef"=w487) -> ()  [unwired: 6 in, 3 out]
                }
                n240 = call <vilib>:"WPI_RobotDriveRefNum Registry Get.vi"("refnum name"="intakeDevice") -> ("RobotDriveDevRef"=w456:T6)  [unwired: 9 in, 1 out]
                n241 = for {
                  N: 50 -> [_]
                  tunnel: w456 -> [w483]
                  tunnel: w455 -> [w479]
                  tunnel: w452 -> [w481]
                  tunnel: [w480] -> w450
                  tunnel: [w479] -> w446
                  stop <- w482 stop-if-true
                  n242 = call <vilib>:"WPI_SwitchGetLimitValue.vi"("SwitchDevRef"=w481) -> ("Switch Pressed"=w482:bool)  [unwired: 8 in, 2 out]
                  n243 = call-poly <vilib>:"WPI_RobotDriveArcadeDrive.vi"("Y axis value"=-0.8, "X axis value"=0.0, "RobotDriveDevRef"=w483) -> ("RobotDriveDevRef"=w480:T6)  [unwired: 6 in, 2 out]
                  n244 = Wait (ms)(milliseconds to wait=u32 50) -> ()  [unwired: 1 out]
                }
                n245 = Tick Count (ms)() -> (millisecond timer value=w447:u32)
                n246 = while {
                  tunnel: w446 -> [w470]
                  tunnel: [w469] -> w445
                  tunnel: w447 -> [w466]
                  stop <- w465 stop-if-true
                  n247 = call "Timeout.vi"("Start Time In"=w466, "Time Limit"=u32 5000) -> ("Timeout"=w465:bool)  [unwired: 8 in, 1 out]
                  n248 = call "Drive Straight Arcade.vi"("Angle robot facing"=0.0) -> ("Arcade drive x"=w463:dbl)  [unwired: 10 in]
                  n249 = call-poly <vilib>:"WPI_RobotDriveArcadeDrive.vi"("Y axis value"=-0.7, "X axis value"=w463, "RobotDriveDevRef"=w470) -> ("RobotDriveDevRef"=w469:T6)  [unwired: 6 in, 2 out]
                  n250 = Wait (ms)(milliseconds to wait=u32 40) -> ()  [unwired: 1 out]
                }
                n251 = for {
                  N: 5 -> [_]
                  tunnel: [w477] -> w449
                  tunnel: w450 -> [w477]
                  n252 = Wait (ms)(milliseconds to wait=u32 50) -> ()  [unwired: 1 out]
                }
                n253 = for {
                  N: 25 -> [_]
                  tunnel: w449 -> [w473]
                  tunnel: [w472] -> _
                  n254 = call-poly <vilib>:"WPI_RobotDriveArcadeDrive.vi"("Y axis value"=0.7, "X axis value"=0.0, "RobotDriveDevRef"=w473) -> ("RobotDriveDevRef"=w472:T6)  [unwired: 6 in, 2 out]
                  n255 = Wait (ms)(milliseconds to wait=u32 50) -> ()  [unwired: 1 out]
                }
              }
            }
          }
          frame 4 {
            # "Turn to the left, so right wheel hits\nedge of rampart. It is easier to go over\nthis way"
            # "Go forward"
            # "RAMPARTS"
            n256 = disable-structure shown="Disabled" {
              disable-tunnel: w496 -> [w501 _]
              frame Disabled {
                # "Raise arm a little"
                n257 = call "Set Arm Position.vi"("RobotDriveDevRef 2"=w501, "Setpoint"=100.0) -> ()  [unwired: 9 in, 1 out]
              }
              frame Enabled {
              }
            }
            n258 = call "Forward For inch.vi"("Angle robot facing"=0.0, "Speed"=-0.65, "Distance"=30.0, "RobotDriveDevRef in"=w496) -> ("RobotDriveDevRef out"=w495:T6)  [unwired: 7 in]
            n259 = call "Turn to degrees.vi"("Speed/Direction"=0.63, "Angle"=-7.0, "RobotDriveDevRef in"=w495) -> ("RobotDriveDevRef out"=w499:T6)  [unwired: 8 in]
            n260 = Tick Count (ms)() -> (millisecond timer value=w491:u32)
            n261 = while {
              tunnel: [w510] -> w500
              tunnel: w499 -> [w506]
              tunnel: w491 -> [w504]
              stop <- w503 stop-if-true
              # "Forward until over"
              n262 = call "Timeout.vi"("Start Time In"=w504, "Time Limit"=u32 4000) -> ("Timeout"=w503:bool)  [unwired: 8 in, 1 out]
              n263 = call "Drive Straight Arcade.vi"("Angle robot facing"=-5.0) -> ("Arcade drive x"=w508:dbl)  [unwired: 10 in]
              n264 = Wait (ms)(milliseconds to wait=u32 20) -> ()  [unwired: 1 out]
              n265 = call-poly <vilib>:"WPI_RobotDriveArcadeDrive.vi"("Y axis value"=-0.68, "X axis value"=w508, "RobotDriveDevRef"=w506) -> ("RobotDriveDevRef"=w510:T6)  [unwired: 6 in, 2 out]
            }
          }
          frame 5 {
            # "MOAT"
            n266 = Tick Count (ms)() -> (millisecond timer value=w512:u32)
            n267 = disable-structure shown="Disabled" {
              disable-tunnel: w513 -> [w515 _]
              frame Disabled {
                # "Raise arm"
                n268 = call "Set Arm Position.vi"("RobotDriveDevRef 2"=w515, "Setpoint"=50.0) -> ()  [unwired: 9 in, 1 out]
              }
              frame Enabled {
              }
            }
            n269 = while {
              tunnel: w513 -> [w523]
              tunnel: [w524] -> w514
              tunnel: w512 -> [w519]
              stop <- w517 stop-if-true
              # "Go forward"
              n270 = call "Timeout.vi"("Start Time In"=w519, "Time Limit"=u32 5000) -> ("Timeout"=w517:bool)  [unwired: 8 in, 1 out]
              n271 = call "Drive Straight Arcade.vi"("Angle robot facing"=0.0) -> ("Arcade drive x"=w520:dbl)  [unwired: 10 in]
              n272 = call-poly <vilib>:"WPI_RobotDriveArcadeDrive.vi"("Y axis value"=-0.75, "X axis value"=w520, "RobotDriveDevRef"=w523) -> ("RobotDriveDevRef"=w524:T6)  [unwired: 6 in, 2 out]
              n273 = Wait (ms)(milliseconds to wait=u32 20) -> ()  [unwired: 1 out]
            }
          }
          frame 6 {
            # "DRAWBRIDGE"
            n274 = Tick Count (ms)() -> (millisecond timer value=w526:u32)
            n275 = while {
              tunnel: w527 -> [w533]
              tunnel: [w534] -> w528
              tunnel: w526 -> [w530]
              stop <- w529 stop-if-true
              n276 = call "Timeout.vi"("Start Time In"=w530, "Time Limit"=u32 4000) -> ("Timeout"=w529:bool)  [unwired: 8 in, 1 out]
              n277 = call-poly <vilib>:"WPI_RobotDriveArcadeDrive.vi"("Y axis value"=-0.6, "X axis value"=0.0 ("Y axis value"), "RobotDriveDevRef"=w533) -> ("RobotDriveDevRef"=w534:T6)  [unwired: 6 in, 2 out]
              n278 = Wait (ms)(milliseconds to wait=u32 20) -> ()  [unwired: 1 out]
            }
          }
          frame 7 {
            # "SALLY PORT"
            n279 = Tick Count (ms)() -> (millisecond timer value=w539:u32)
            n280 = while {
              tunnel: w538 -> [w544]
              tunnel: [w545] -> w537
              tunnel: w539 -> [w541]
              stop <- w540 stop-if-true
              n281 = call "Timeout.vi"("Start Time In"=w541, "Time Limit"=u32 4000) -> ("Timeout"=w540:bool)  [unwired: 8 in, 1 out]
              n282 = call-poly <vilib>:"WPI_RobotDriveArcadeDrive.vi"("Y axis value"=-0.6, "X axis value"=0.0 ("Y axis value"), "RobotDriveDevRef"=w544) -> ("RobotDriveDevRef"=w545:T6)  [unwired: 6 in, 2 out]
              n283 = Wait (ms)(milliseconds to wait=u32 20) -> ()  [unwired: 1 out]
            }
          }
          frame 8 {
            # "ROCK WALL"
            # "Forward fast\nto save time"
            n284 = call "Forward For inch.vi"("Angle robot facing"=0.0, "Speed"=-0.85, "Distance"=35.0, "RobotDriveDevRef in"=w553) -> ("RobotDriveDevRef out"=w552:T6)  [unwired: 7 in]
            n285 = disable-structure shown="Disabled" {
              disable-tunnel: w553 -> [w555 _]
              frame Disabled {
                n286 = call "Set Arm Position.vi"("RobotDriveDevRef 2"=w555, "Setpoint"=50.0) -> ()  [unwired: 9 in, 1 out]
              }
              frame Enabled {
              }
            }
            n287 = Tick Count (ms)() -> (millisecond timer value=w548:u32)
            n288 = while {
              tunnel: w552 -> [w563]
              tunnel: [w564] -> w554
              tunnel: w548 -> [w557]
              stop <- w558 stop-if-true
              # "Forward"
              n289 = call "Timeout.vi"("Start Time In"=w557, "Time Limit"=u32 3500) -> ("Timeout"=w558:bool)  [unwired: 8 in, 1 out]
              n290 = call "Drive Straight Arcade.vi"("Angle robot facing"=0.0) -> ("Arcade drive x"=w561:dbl)  [unwired: 10 in]
              n291 = call-poly <vilib>:"WPI_RobotDriveArcadeDrive.vi"("Y axis value"=-0.65, "X axis value"=w561, "RobotDriveDevRef"=w563) -> ("RobotDriveDevRef"=w564:T6)  [unwired: 6 in, 2 out]
              n292 = Wait (ms)(milliseconds to wait=u32 20) -> ()  [unwired: 1 out]
            }
          }
          frame 9 {
            n293 = Tick Count (ms)() -> (millisecond timer value=w567:u32)
            n294 = disable-structure shown="Disabled" {
              disable-tunnel: w568 -> [w569 _]
              frame Disabled {
                # "Arm up"
                # "ROUGH TERRAIN"
                n295 = call "Set Arm Position.vi"("RobotDriveDevRef 2"=w569, "Setpoint"=100.0) -> ()  [unwired: 9 in, 1 out]
              }
              frame Enabled {
              }
            }
            n296 = while {
              tunnel: w568 -> [w577]
              tunnel: [w578] -> w566
              tunnel: w567 -> [w572]
              stop <- w571 stop-if-true
              # "Go forward"
              n297 = call "Timeout.vi"("Start Time In"=w572, "Time Limit"=u32 4000) -> ("Timeout"=w571:bool)  [unwired: 8 in, 1 out]
              n298 = call "Drive Straight Arcade.vi"("Angle robot facing"=0.0) -> ("Arcade drive x"=w575:dbl)  [unwired: 10 in]
              n299 = Wait (ms)(milliseconds to wait=u32 20) -> ()  [unwired: 1 out]
              n300 = call-poly <vilib>:"WPI_RobotDriveArcadeDrive.vi"("Y axis value"=-0.65, "X axis value"=w575, "RobotDriveDevRef"=w577) -> ("RobotDriveDevRef"=w578:T6)  [unwired: 6 in, 2 out]
            }
          }
        }
        n301 = flat-sequence {
          tunnel: w234 -> [_]
          frame #0 {
            n302 = local write "Stop Wheel Loop"(TRUE) -> ()
          }
        }
        n303 = call-poly <vilib>:"NT Read Value.vi"("Name"="Shoot") -> ("Boolean"=w225:bool)  [unwired: 9 in, 1 out]
        n304 = call-poly <vilib>:"NT Read Value.vi"("Name"="Defense Position") -> ("Numeric"=w224:dbl)  [unwired: 9 in, 1 out]
        n305 = case shown="True" w225 {
          tunnel: w224 -> [_ w668]
          tunnel: w232 -> [w580 w667]
          tunnel: w227 -> [_ w665]
          tunnel: w223 -> [_ w664]
          frame False {
            n306 = call-poly <vilib>:"NT Read Value.vi"("Name"="Cross Back") -> ("Boolean"=w582:bool)  [unwired: 9 in, 1 out]
            n307 = case shown="False" w582 {
              tunnel: w580 -> [_ w587]
              frame False {
                n308 = call-poly <vilib>:"NT Write Value.vi"("Numeric"=3.0, "Name"="Template") -> ()  [unwired: 9 in, 1 out]
              }
              frame True {
                n309 = Tick Count (ms)() -> (millisecond timer value=w586:u32)
                n310 = while {
                  tunnel: w586 -> [w593]
                  tunnel: [w590] -> w585
                  stop <- w592 stop-if-true
                  w590 = u32 20 ("milliseconds to wait")
                  n311 = Wait (ms)(milliseconds to wait=w590) -> ()  [unwired: 1 out]
                  n312 = call "Timeout.vi"("Start Time In"=w593, "Time Limit"=u32 500 ("milliseconds to wait")) -> ("Timeout"=w592:bool)  [unwired: 8 in, 1 out]
                }
                n313 = call-poly <vilib>:"NT Read Value.vi"("Name"="Defense") -> ("Numeric"=w588:dbl)  [unwired: 9 in, 1 out]
                n314 = case shown="1" w588 {
                  tunnel: w587 -> [_ w595 _ _ w601 w611 w622 w632 w642 w653]
                  tunnel: w585 -> [_ _ _ _ _ _ _ _ _ _]
                  frame 0, Default {
                  }
                  frame 1 {
                    # "LOW BAR"
                    # "in front of outer works\nto neutral zone"
                    # "drive forward from castle \nwall to outer works"
                    n315 = call "Set Arm Position.vi"("RobotDriveDevRef 2"=w595, "Speed"=0.8, "Setpoint"=600.0) -> ("RobotDriveDevRef"=w594:T6)  [unwired: 8 in]
                    n316 = call "Forward For inch.vi"("Angle robot facing"=0.0, "Speed"=-0.65, "Distance"=192.0, "RobotDriveDevRef in"=w594) -> ()  [unwired: 7 in, 1 out]
                  }
                  frame 2 {
                    # "PORTCULLIS"
                    # "NOT WORTH IT"
                    # "NO"
                  }
                  frame 3 {
                    # "CDF"
                    # "NOT WORTH IT EITHER, CROSSING IS GOOD ENOUGH"
                  }
                  frame 4 {
                    # "RAMPARTS"
                    n317 = Tick Count (ms)() -> (millisecond timer value=w602:u32)
                    n318 = while {
                      tunnel: w602 -> [w605]
                      tunnel: w601 -> [w603]
                      stop <- w604 stop-if-true
                      # "Forward until over"
                      n319 = call "Timeout.vi"("Start Time In"=w605, "Time Limit"=u32 3000) -> ("Timeout"=w604:bool)  [unwired: 8 in, 1 out]
                      n320 = call "Drive Straight Arcade.vi"("Angle robot facing"=-5.0) -> ("Arcade drive x"=w608:dbl)  [unwired: 10 in]
                      n321 = Wait (ms)(milliseconds to wait=u32 20) -> ()  [unwired: 1 out]
                      n322 = call-poly <vilib>:"WPI_RobotDriveArcadeDrive.vi"("Y axis value"=0.68, "X axis value"=w608, "RobotDriveDevRef"=w603) -> ()  [unwired: 6 in, 3 out]
                    }
                  }
                  frame 5 {
                    # "MOAT"
                    n323 = Tick Count (ms)() -> (millisecond timer value=w612:u32)
                    n324 = while {
                      tunnel: w611 -> [w619]
                      tunnel: [w620] -> _
                      tunnel: w612 -> [w615]
                      stop <- w613 stop-if-true
                      # "Go forward"
                      n325 = call "Timeout.vi"("Start Time In"=w615, "Time Limit"=u32 4000) -> ("Timeout"=w613:bool)  [unwired: 8 in, 1 out]
                      n326 = call "Drive Straight Arcade.vi"("Angle robot facing"=0.0) -> ("Arcade drive x"=w616:dbl)  [unwired: 10 in]
                      n327 = call-poly <vilib>:"WPI_RobotDriveArcadeDrive.vi"("Y axis value"=0.75, "X axis value"=w616, "RobotDriveDevRef"=w619) -> ("RobotDriveDevRef"=w620:T6)  [unwired: 6 in, 2 out]
                      n328 = Wait (ms)(milliseconds to wait=u32 20) -> ()  [unwired: 1 out]
                    }
                  }
                  frame 6 {
                    # "DRAWBRIDGE"
                    n329 = Tick Count (ms)() -> (millisecond timer value=w623:u32)
                    n330 = while {
                      tunnel: w622 -> [w628]
                      tunnel: [w629] -> _
                      tunnel: w623 -> [w625]
                      stop <- w624 stop-if-true
                      n331 = call "Timeout.vi"("Start Time In"=w625, "Time Limit"=u32 3000) -> ("Timeout"=w624:bool)  [unwired: 8 in, 1 out]
                      n332 = call-poly <vilib>:"WPI_RobotDriveArcadeDrive.vi"("Y axis value"=0.6, "X axis value"=0.0 ("Y axis value"), "RobotDriveDevRef"=w628) -> ("RobotDriveDevRef"=w629:T6)  [unwired: 6 in, 2 out]
                      n333 = Wait (ms)(milliseconds to wait=u32 20) -> ()  [unwired: 1 out]
                    }
                  }
                  frame 7 {
                    # "SALLY PORT"
                    n334 = Tick Count (ms)() -> (millisecond timer value=w633:u32)
                    n335 = while {
                      tunnel: w632 -> [w638]
                      tunnel: [w639] -> _
                      tunnel: w633 -> [w635]
                      stop <- w634 stop-if-true
                      n336 = call "Timeout.vi"("Start Time In"=w635, "Time Limit"=u32 3000) -> ("Timeout"=w634:bool)  [unwired: 8 in, 1 out]
                      n337 = call-poly <vilib>:"WPI_RobotDriveArcadeDrive.vi"("Y axis value"=0.6, "X axis value"=0.0 ("Y axis value"), "RobotDriveDevRef"=w638) -> ("RobotDriveDevRef"=w639:T6)  [unwired: 6 in, 2 out]
                      n338 = Wait (ms)(milliseconds to wait=u32 20) -> ()  [unwired: 1 out]
                    }
                  }
                  frame 8 {
                    # "ROCK WALL"
                    n339 = Tick Count (ms)() -> (millisecond timer value=w643:u32)
                    n340 = while {
                      tunnel: w642 -> [w650]
                      tunnel: [w651] -> _
                      tunnel: w643 -> [w644]
                      stop <- w645 stop-if-true
                      # "Forward"
                      n341 = call "Timeout.vi"("Start Time In"=w644, "Time Limit"=u32 2500) -> ("Timeout"=w645:bool)  [unwired: 8 in, 1 out]
                      n342 = call "Drive Straight Arcade.vi"("Angle robot facing"=0.0) -> ("Arcade drive x"=w648:dbl)  [unwired: 10 in]
                      n343 = call-poly <vilib>:"WPI_RobotDriveArcadeDrive.vi"("Y axis value"=0.65, "X axis value"=w648, "RobotDriveDevRef"=w650) -> ("RobotDriveDevRef"=w651:T6)  [unwired: 6 in, 2 out]
                      n344 = Wait (ms)(milliseconds to wait=u32 20) -> ()  [unwired: 1 out]
                    }
                  }
                  frame 9 {
                    n345 = Tick Count (ms)() -> (millisecond timer value=w654:u32)
                    n346 = while {
                      tunnel: [w662] -> _
                      tunnel: w654 -> [w657]
                      tunnel: w653 -> [w655]
                      stop <- w656 stop-if-true
                      # "Go forward"
                      n347 = call "Timeout.vi"("Start Time In"=w657, "Time Limit"=u32 4000) -> ("Timeout"=w656:bool)  [unwired: 8 in, 1 out]
                      n348 = call "Drive Straight Arcade.vi"("Angle robot facing"=0.0) -> ("Arcade drive x"=w660:dbl)  [unwired: 10 in]
                      n349 = Wait (ms)(milliseconds to wait=u32 20) -> ()  [unwired: 1 out]
                      n350 = call-poly <vilib>:"WPI_RobotDriveArcadeDrive.vi"("Y axis value"=0.65, "X axis value"=w660, "RobotDriveDevRef"=w655) -> ("RobotDriveDevRef"=w662:T6)  [unwired: 6 in, 2 out]
                    }
                  }
                }
              }
            }
          }
          frame True {
            n351 = case shown="4" w668 {
              tunnel: w667 -> [_ w692 w788 w887 w978 w992]
              tunnel: w664 -> [_ w683 w779 w897 _ w993]
              frame 0, Default {
              }
              frame 1 {
                # "disabled case for driving to wall\n at an angle"
                # "disabled case for driving to wall\nat an angle"
                # "Raise arm so it doesn't\ndrag on ground"
                # "This ensures that the intake wheels spit out the boulder with\none second left in auto, no matter if the other\nactions (the last turning part is our real concern) finish."
                # "Lower arm"
                # "Shoot"
                n352 = disable-structure shown="Disabled" {
                  disable-tunnel: w692 -> [w738 _]
                  frame Disabled {
                    n353 = call "Set Arm Position.vi"("RobotDriveDevRef 2"=w738, "Speed"=0.8, "Setpoint"=480.0) -> ()  [unwired: 8 in, 1 out]
                  }
                  frame Enabled {
                  }
                }
                n354 = call <vilib>:"WPI_AccelerometerRefNum Registry Get.vi"("refnum name"="accel") -> ("AccelerometerDevRef"=w697:T14)  [unwired: 9 in, 1 out]
                n355 = while {
                  tunnel: w683 -> [w712]
                  tunnel: [w711] -> w682
                  stop <- w711 stop-if-true
                  n356 = call "Timeout.vi"("Start Time In"=w712, "Time Limit"=u32 14000) -> ("Timeout"=w711:bool)  [unwired: 8 in, 1 out]
                  n357 = Wait (ms)(milliseconds to wait=u32 300) -> ()  [unwired: 1 out]
                }
                n358 = Tick Count (ms)() -> (millisecond timer value=w689:u32)
                n359 = while {
                  tunnel: w697 -> [w758]
                  tunnel: w692 -> [w750]
                  tunnel: [w749] -> w686
                  tunnel: [w748] -> _
                  tunnel: w689 -> [w745]
                  stop <- w747 stop-if-true
                  n360 = disable-structure shown="Enabled" {
                    disable-tunnel: [w761 0.0 ("X axis value")] -> w743
                    disable-tunnel: [u32 10000 ("Time Limit") u32 10000 ("Time Limit")] -> w742
                    frame Enabled {
                      n361 = call "Drive Straight Arcade.vi"("Angle robot facing"=10.0) -> ("Arcade drive x"=w761:dbl)  [unwired: 10 in]
                    }
                    frame Disabled {
                    }
                  }
                  n362 = call <vilib>:"WPI_AccelerometerGetAcceleration.vi"("AccelerometerDevRef"=w758) -> ("Accelerations"=w757:T20, "AccelerometerDevRef"=w748:T14)  [unwired: 8 in, 1 out]
                  n363 = call "Timeout.vi"("Start Time In"=w745, "Time Limit"=w742) -> ("Timeout"=w744:bool)  [unwired: 8 in, 1 out]
                  n364 = Unbundle By Name(w757) -> ("Y-Axis"=w753:dbl)
                  n365 = In Range and Coerce(upper limit=0.8, x=w753, lower limit=-0.8) -> (In Range?=w754:bool)  [unwired: 1 out]
                  n366 = Not(x=w754) -> (.not. x?=w746:bool)
                  n367 = call-poly <vilib>:"WPI_RobotDriveArcadeDrive.vi"("Y axis value"=0.65, "X axis value"=w743, "RobotDriveDevRef"=w750) -> ("RobotDriveDevRef"=w749:T6)  [unwired: 6 in, 2 out]
                  n368 = Or(x=w746, y=w744) -> (x .or. y?=w747:bool)
                  n369 = Wait (ms)(milliseconds to wait=u32 20) -> ()  [unwired: 1 out]
                }
                n370 = disable-structure shown="Disabled" {
                  frame Disabled {
                    n371 = call "Turn And Shoot.vi"("Turning Angle"=-95.0) -> ()  [unwired: 11 in]
                  }
                  frame Enabled {
                  }
                }
                n372 = for {
                  N: 1 -> [_]
                  tunnel: [w731] -> w685
                  tunnel: w686 -> [w731]
                  n373 = Wait (ms)(milliseconds to wait=u32 350) -> ()  [unwired: 1 out]
                }
                n374 = call <vilib>:"WPI_RobotDriveRefNum Registry Get.vi"("refnum name"="intakeDevice") -> ("RobotDriveDevRef"=w674:T6)  [unwired: 9 in, 1 out]
                n375 = call "Forward For inch.vi"("Angle robot facing"=0.0, "Speed"=-0.6, "Distance"=2.0, "RobotDriveDevRef in"=w685) -> ("RobotDriveDevRef out"=w672:T6)  [unwired: 7 in]
                n376 = for {
                  N: 40 -> [_]
                  tunnel: w674 -> [w705]
                  tunnel: w672 -> [_]
                  tunnel: [w703] -> w669
                  n377 = call-poly <vilib>:"WPI_RobotDriveArcadeDrive.vi"("Y axis value"=0.6, "X axis value"=0.0, "RobotDriveDevRef"=w705) -> ("RobotDriveDevRef"=w703:T6)  [unwired: 6 in, 2 out]
                  n378 = Wait (ms)(milliseconds to wait=u32 20) -> ()  [unwired: 1 out]
                }
                n379 = disable-structure shown="Enabled" {
                  disable-tunnel: [-100.0 ("Angle") -90.0 ("Angle")] -> w677
                  frame Disabled {
                  }
                  frame Enabled {
                  }
                }
                n380 = call "Turn to degrees.vi"("Speed/Direction"=-0.9, "Angle"=w677, "RobotDriveDevRef in"=w672) -> ("RobotDriveDevRef out"=w670:T6)  [unwired: 8 in]
                n381 = call-poly <vilib>:"NT Write Value.vi"("Numeric"=3.0, "Name"="Template") -> ()  [unwired: 9 in, 1 out]
                n382 = for {
                  N: 30 -> [_]
                  tunnel: w669 -> [w700]
                  tunnel: w670 -> [_]
                  n383 = call-poly <vilib>:"WPI_RobotDriveArcadeDrive.vi"("Y axis value"=-0.5, "X axis value"=0.0, "RobotDriveDevRef"=w700) -> ()  [unwired: 6 in, 3 out]
                  n384 = Wait (ms)(milliseconds to wait=u32 20) -> ()  [unwired: 1 out]
                }
                n385 = disable-structure shown="Enabled" {
                  disable-tunnel: w670 -> [w715 w720]
                  disable-tunnel: [w714 w719] -> w684
                  frame Disabled {
                    n386 = call "Forward For inch.vi"("Angle robot facing"=-90.0, "Speed"=-0.6, "Distance"=72.0, "RobotDriveDevRef in"=w715) -> ("RobotDriveDevRef out"=w714:T6)  [unwired: 7 in]
                  }
                  frame Enabled {
                    n387 = disable-structure shown="Disabled" {
                      disable-tunnel: w720 -> [w724 _]
                      frame Disabled {
                        n388 = call "Set Arm Position.vi"("RobotDriveDevRef 2"=w724, "Speed"=0.8, "Setpoint"=550.0) -> ()  [unwired: 8 in, 1 out]
                      }
                      frame Enabled {
                      }
                    }
                    n389 = for {
                      N: 50 -> [_]
                      tunnel: w720 -> [w728]
                      tunnel: [w727] -> w719
                      n390 = call "Drive Straight Arcade.vi"("Angle robot facing"=-90.0) -> ("Arcade drive x"=w725:dbl)  [unwired: 10 in]
                      n391 = Wait (ms)(milliseconds to wait=u32 50) -> ()  [unwired: 1 out]
                      n392 = call-poly <vilib>:"WPI_RobotDriveArcadeDrive.vi"("Y axis value"=-0.65, "X axis value"=w725, "RobotDriveDevRef"=w728) -> ("RobotDriveDevRef"=w727:T6)  [unwired: 6 in, 2 out]
                    }
                  }
                }
                n393 = call "Turn to degrees.vi"("Speed/Direction"=-0.7, "Angle"=-115.0, "RobotDriveDevRef in"=w684) -> ("RobotDriveDevRef out"=w676:T6)  [unwired: 8 in]
                n394 = disable-structure shown="Enabled" {
                  disable-tunnel: w676 -> [w733 _]
                  frame Disabled {
                    n395 = call "Set Arm Position.vi"("RobotDriveDevRef 2"=w733, "Speed"=0.9, "Setpoint"=620.0) -> ()  [unwired: 8 in, 1 out]
                  }
                  frame Enabled {
                  }
                }
                n396 = call <vilib>:"WPI_MotorControlRefNum Registry Get.vi"("refnum name"="intakeWheels") -> ("MotorControlDevRef"=w694:T7)  [unwired: 9 in, 1 out]
                n397 = for {
                  N: 20 -> [_]
                  tunnel: w694 -> [w741]
                  tunnel: w682 -> [_]
                  n398 = Wait (ms)(milliseconds to wait=u32 50) -> ()  [unwired: 1 out]
                  n399 = call <vilib>:"WPI_MotorControlSetOutput.vi"("Output"=-1.0, "MotorControlDevRef"=w741) -> ()  [unwired: 7 in, 3 out]
                }
              }
              frame 5 {
                # "may be too much"
                # "Defense position 5"
                # "This ensures that the intake wheels spit out the boulder with one second left in auto, no matter if the other\nactions (the last turning part is our real concern) finish."
                # "Lower arm"
                # "Shoot"
                n400 = disable-structure shown="Disabled" {
                  disable-tunnel: w788 -> [w846 _]
                  frame Disabled {
                    n401 = call "Set Arm Position.vi"("RobotDriveDevRef 2"=w846, "Speed"=0.8, "Setpoint"=480.0) -> ()  [unwired: 8 in, 1 out]
                  }
                  frame Enabled {
                  }
                }
                n402 = call <vilib>:"WPI_AccelerometerRefNum Registry Get.vi"("refnum name"="accel") -> ("AccelerometerDevRef"=w793:T14)  [unwired: 9 in, 1 out]
                n403 = while {
                  tunnel: w779 -> [w820]
                  tunnel: [w819] -> w778
                  stop <- w819 stop-if-true
                  n404 = call "Timeout.vi"("Start Time In"=w820, "Time Limit"=u32 14000) -> ("Timeout"=w819:bool)  [unwired: 8 in, 1 out]
                  n405 = Wait (ms)(milliseconds to wait=u32 300) -> ()  [unwired: 1 out]
                }
                n406 = Tick Count (ms)() -> (millisecond timer value=w785:u32)
                n407 = while {
                  tunnel: w793 -> [w866]
                  tunnel: w788 -> [w858]
                  tunnel: [w857] -> w782
                  tunnel: [w856] -> _
                  tunnel: w785 -> [w853]
                  stop <- w855 stop-if-true
                  n408 = disable-structure shown="Enabled" {
                    disable-tunnel: [w869 0.0 ("X axis value")] -> w851
                    disable-tunnel: [u32 10000 ("Time Limit") u32 10000 ("Time Limit")] -> w850
                    frame Enabled {
                      n409 = call "Drive Straight Arcade.vi"("Angle robot facing"=1.0) -> ("Arcade drive x"=w869:dbl)  [unwired: 10 in]
                    }
                    frame Disabled {
                    }
                  }
                  n410 = call <vilib>:"WPI_AccelerometerGetAcceleration.vi"("AccelerometerDevRef"=w866) -> ("Accelerations"=w865:T20, "AccelerometerDevRef"=w856:T14)  [unwired: 8 in, 1 out]
                  n411 = call "Timeout.vi"("Start Time In"=w853, "Time Limit"=w850) -> ("Timeout"=w852:bool)  [unwired: 8 in, 1 out]
                  n412 = Unbundle By Name(w865) -> ("Y-Axis"=w861:dbl)
                  n413 = In Range and Coerce(upper limit=0.8, x=w861, lower limit=-0.8) -> (In Range?=w862:bool)  [unwired: 1 out]
                  n414 = Not(x=w862) -> (.not. x?=w854:bool)
                  n415 = call-poly <vilib>:"WPI_RobotDriveArcadeDrive.vi"("Y axis value"=-0.65, "X axis value"=w851, "RobotDriveDevRef"=w858) -> ("RobotDriveDevRef"=w857:T6)  [unwired: 6 in, 2 out]
                  n416 = Or(x=w854, y=w852) -> (x .or. y?=w855:bool)
                  n417 = Wait (ms)(milliseconds to wait=u32 20) -> ()  [unwired: 1 out]
                }
                n418 = disable-structure shown="Disabled" {
                  frame Disabled {
                    n419 = call "Turn And Shoot.vi"("Turning Angle"=-95.0) -> ()  [unwired: 11 in]
                  }
                  frame Enabled {
                  }
                }
                n420 = for {
                  N: 1 -> [_]
                  tunnel: [w839] -> w781
                  tunnel: w782 -> [w839]
                  n421 = Wait (ms)(milliseconds to wait=u32 350) -> ()  [unwired: 1 out]
                }
                n422 = call <vilib>:"WPI_RobotDriveRefNum Registry Get.vi"("refnum name"="intakeDevice") -> ("RobotDriveDevRef"=w772:T6)  [unwired: 9 in, 1 out]
                n423 = call <vilib>:"WPI_SwitchRefNum Registry Get.vi"("refnum name"="mechanismSwitch") -> ("SwitchDevRef"=w768:T12)  [unwired: 9 in, 1 out]
                n424 = call <vilib>:"WPI_GyroRefNum Registry Get.vi"("refnum name"="Gyro") -> ("GyroDevRef"=w765:T2)  [unwired: 9 in, 1 out]
                n425 = call "Forward For inch.vi"("Angle robot facing"=0.0, "Speed"=0.6, "Distance"=-6.0, "RobotDriveDevRef in"=w781) -> ("RobotDriveDevRef out"=w770:T6)  [unwired: 7 in]
                n426 = for {
                  N: 175 -> [_]
                  tunnel: w772 -> [w815]
                  tunnel: w770 -> [_]
                  tunnel: [w813] -> _
                  tunnel: w768 -> [w811]
                  stop <- w812 stop-if-true
                  n427 = call <vilib>:"WPI_SwitchGetLimitValue.vi"("SwitchDevRef"=w811) -> ("Switch Pressed"=w812:bool)  [unwired: 8 in, 2 out]
                  n428 = call-poly <vilib>:"WPI_RobotDriveArcadeDrive.vi"("Y axis value"=-0.7, "X axis value"=0.0, "RobotDriveDevRef"=w815) -> ("RobotDriveDevRef"=w813:T6)  [unwired: 6 in, 2 out]
                  n429 = Wait (ms)(milliseconds to wait=u32 20) -> ()  [unwired: 1 out]
                }
                n430 = disable-structure shown="Enabled" {
                  disable-tunnel: w770 -> [w796 w801]
                  disable-tunnel: [w795 w800] -> w767
                  disable-tunnel: w765 -> [_ w799]
                  frame Disabled {
                    n431 = call "Turn to degrees.vi"("Speed/Direction"=-1.0, "Angle"=-70.0, "RobotDriveDevRef in"=w796) -> ("RobotDriveDevRef out"=w795:T6)  [unwired: 8 in]
                  }
                  frame Enabled {
                    n432 = while {
                      tunnel: w801 -> [w810]
                      tunnel: [w809] -> w800
                      tunnel: w799 -> [w806]
                      stop <- w803 stop-if-true
                      n433 = call <vilib>:"WPI_GyroGetAngle.vi"("GyroDevRef"=w806) -> ("Angle"=w805:dbl)  [unwired: 6 in, 4 out]
                      n434 = Wait (ms)(milliseconds to wait=u32 30) -> ()  [unwired: 1 out]
                      n435 = call-poly <vilib>:"WPI_RobotDriveArcadeDrive.vi"("Y axis value"=0.0, "X axis value"=-1.0, "RobotDriveDevRef"=w810) -> ("RobotDriveDevRef"=w809:T6)  [unwired: 6 in, 2 out]
                      n436 = Less Or Equal?(x=w805, y=-70.0) -> (x <= y?=w803:bool)
                    }
                  }
                }
                n437 = call-poly <vilib>:"NT Write Value.vi"("Numeric"=3.0, "Name"="Template") -> ()  [unwired: 9 in, 1 out]
                n438 = disable-structure shown="Enabled" {
                  disable-tunnel: w767 -> [w823 w828]
                  disable-tunnel: [w822 w827] -> w780
                  frame Disabled {
                    n439 = call "Forward For inch.vi"("Angle robot facing"=-90.0, "Speed"=-0.6, "Distance"=72.0, "RobotDriveDevRef in"=w823) -> ("RobotDriveDevRef out"=w822:T6)  [unwired: 7 in]
                  }
                  frame Enabled {
                    n440 = disable-structure shown="Disabled" {
                      disable-tunnel: w828 -> [w832 _]
                      frame Disabled {
                        n441 = call "Set Arm Position.vi"("RobotDriveDevRef 2"=w832, "Speed"=0.8, "Setpoint"=550.0) -> ()  [unwired: 8 in, 1 out]
                      }
                      frame Enabled {
                      }
                    }
                    n442 = for {
                      N: 20 -> [_]
                      tunnel: w828 -> [w836]
                      tunnel: [w835] -> w827
                      n443 = call "Drive Straight Arcade.vi"("Angle robot facing"=-80.0) -> ("Arcade drive x"=w833:dbl)  [unwired: 10 in]
                      n444 = Wait (ms)(milliseconds to wait=u32 50) -> ()  [unwired: 1 out]
                      n445 = call-poly <vilib>:"WPI_RobotDriveArcadeDrive.vi"("Y axis value"=-0.55, "X axis value"=w833, "RobotDriveDevRef"=w836) -> ("RobotDriveDevRef"=w835:T6)  [unwired: 6 in, 2 out]
                    }
                  }
                }
                n446 = call "Turn to degrees.vi"("Speed/Direction"=0.7, "Angle"=-65.0, "RobotDriveDevRef in"=w780) -> ("RobotDriveDevRef out"=w774:T6)  [unwired: 8 in]
                n447 = disable-structure shown="Enabled" {
                  disable-tunnel: w774 -> [w841 _]
                  frame Disabled {
                    n448 = call "Set Arm Position.vi"("RobotDriveDevRef 2"=w841, "Speed"=0.9, "Setpoint"=620.0) -> ()  [unwired: 8 in, 1 out]
                  }
                  frame Enabled {
                  }
                }
                n449 = call <vilib>:"WPI_MotorControlRefNum Registry Get.vi"("refnum name"="intakeWheels") -> ("MotorControlDevRef"=w790:T7)  [unwired: 9 in, 1 out]
                n450 = for {
                  N: 20 -> [_]
                  tunnel: w790 -> [w849]
                  tunnel: w778 -> [_]
                  tunnel: w767 -> [_]
                  n451 = Wait (ms)(milliseconds to wait=u32 50) -> ()  [unwired: 1 out]
                  n452 = call <vilib>:"WPI_MotorControlSetOutput.vi"("Output"=-1.0, "MotorControlDevRef"=w849) -> ()  [unwired: 7 in, 3 out]
                }
              }
              frame 4 {
                w882 = 75.0 ("Angle")
                # "may be too much"
                # "Turn and align as if coming out\nof defense 5"
                # "Defense position 4"
                # "disabled case for driving to wall\n at an angle"
                # "Raise arm so it doesn't\ndrag on ground"
                # "This ensures that the intake wheels spit out the boulder with one second left in auto, no matter if the other\nactions (the last turning part is our real concern) finish."
                # "Lower arm"
                # "Shoot"
                n453 = disable-structure shown="Disabled" {
                  disable-tunnel: w887 -> [w949 _]
                  frame Disabled {
                    n454 = call "Set Arm Position.vi"("RobotDriveDevRef 2"=w949, "Speed"=0.8, "Setpoint"=480.0) -> ()  [unwired: 8 in, 1 out]
                  }
                  frame Enabled {
                  }
                }
                n455 = call "Turn to degrees.vi"("Speed/Direction"=0.75, "Angle"=w882, "RobotDriveDevRef in"=w887) -> ("RobotDriveDevRef out"=w889:T6)  [unwired: 8 in]
                n456 = call "Forward For inch.vi"("Angle robot facing"=w882, "Speed"=-0.7, "Distance"=51.0, "RobotDriveDevRef in"=w889) -> ("RobotDriveDevRef out"=w888:T6)  [unwired: 7 in]
                n457 = call <vilib>:"WPI_AccelerometerRefNum Registry Get.vi"("refnum name"="accel") -> ("AccelerometerDevRef"=w910:T14)  [unwired: 9 in, 1 out]
                n458 = while {
                  tunnel: w897 -> [w923]
                  tunnel: [w922] -> w896
                  stop <- w922 stop-if-true
                  n459 = call "Timeout.vi"("Start Time In"=w923, "Time Limit"=u32 14000) -> ("Timeout"=w922:bool)  [unwired: 8 in, 1 out]
                  n460 = Wait (ms)(milliseconds to wait=u32 300) -> ()  [unwired: 1 out]
                }
                n461 = Tick Count (ms)() -> (millisecond timer value=w903:u32)
                n462 = call "Turn to degrees.vi"("Speed/Direction"=-0.75, "Angle"=0.0, "RobotDriveDevRef in"=w888) -> ("RobotDriveDevRef out"=w886:T6)  [unwired: 8 in]
                n463 = while {
                  tunnel: w910 -> [w969]
                  tunnel: w886 -> [w961]
                  tunnel: [w960] -> w900
                  tunnel: [w959] -> _
                  tunnel: w903 -> [w956]
                  stop <- w958 stop-if-true
                  n464 = disable-structure shown="Enabled" {
                    disable-tunnel: [w972 0.0 ("X axis value")] -> w954
                    disable-tunnel: [u32 15000 ("Time Limit") u32 10000 ("Time Limit")] -> w953
                    frame Enabled {
                      n465 = call "Drive Straight Arcade.vi"("Angle robot facing"=3.0) -> ("Arcade drive x"=w972:dbl)  [unwired: 10 in]
                    }
                    frame Disabled {
                    }
                  }
                  n466 = call <vilib>:"WPI_AccelerometerGetAcceleration.vi"("AccelerometerDevRef"=w969) -> ("Accelerations"=w968:T20, "AccelerometerDevRef"=w959:T14)  [unwired: 8 in, 1 out]
                  n467 = call "Timeout.vi"("Start Time In"=w956, "Time Limit"=w953) -> ("Timeout"=w955:bool)  [unwired: 8 in, 1 out]
                  n468 = Unbundle By Name(w968) -> ("Y-Axis"=w964:dbl)
                  n469 = In Range and Coerce(upper limit=0.8, x=w964, lower limit=-0.8) -> (In Range?=w965:bool)  [unwired: 1 out]
                  n470 = Not(x=w965) -> (.not. x?=w957:bool)
                  n471 = call-poly <vilib>:"WPI_RobotDriveArcadeDrive.vi"("Y axis value"=-0.65, "X axis value"=w954, "RobotDriveDevRef"=w961) -> ("RobotDriveDevRef"=w960:T6)  [unwired: 6 in, 2 out]
                  n472 = Or(x=w957, y=w955) -> (x .or. y?=w958:bool)
                  n473 = Wait (ms)(milliseconds to wait=u32 20) -> ()  [unwired: 1 out]
                }
                n474 = disable-structure shown="Disabled" {
                  frame Disabled {
                    n475 = call "Turn And Shoot.vi"("Turning Angle"=-95.0) -> ()  [unwired: 11 in]
                  }
                  frame Enabled {
                  }
                }
                n476 = for {
                  N: 1 -> [_]
                  tunnel: [w942] -> w899
                  tunnel: w900 -> [w942]
                  n477 = Wait (ms)(milliseconds to wait=u32 350) -> ()  [unwired: 1 out]
                }
                n478 = call <vilib>:"WPI_RobotDriveRefNum Registry Get.vi"("refnum name"="intakeDevice") -> ("RobotDriveDevRef"=w878:T6)  [unwired: 9 in, 1 out]
                n479 = call <vilib>:"WPI_SwitchRefNum Registry Get.vi"("refnum name"="mechanismSwitch") -> ("SwitchDevRef"=w875:T12)  [unwired: 9 in, 1 out]
                n480 = call "Forward For inch.vi"("Angle robot facing"=0.0, "Speed"=0.6, "Distance"=-6.0, "RobotDriveDevRef in"=w899) -> ("RobotDriveDevRef out"=w874:T6)  [unwired: 7 in]
                n481 = for {
                  N: 175 -> [_]
                  tunnel: w878 -> [w916]
                  tunnel: [w914] -> _
                  tunnel: w875 -> [w912]
                  tunnel: w874 -> [_]
                  stop <- w913 stop-if-true
                  n482 = call <vilib>:"WPI_SwitchGetLimitValue.vi"("SwitchDevRef"=w912) -> ("Switch Pressed"=w913:bool)  [unwired: 8 in, 2 out]
                  n483 = call-poly <vilib>:"WPI_RobotDriveArcadeDrive.vi"("Y axis value"=-0.7, "X axis value"=0.0, "RobotDriveDevRef"=w916) -> ("RobotDriveDevRef"=w914:T6)  [unwired: 6 in, 2 out]
                  n484 = Wait (ms)(milliseconds to wait=u32 20) -> ()  [unwired: 1 out]
                }
                n485 = disable-structure shown="Enabled" {
                  disable-tunnel: [-100.0 ("Angle") -70.0 ("Angle")] -> w891
                  frame Disabled {
                  }
                  frame Enabled {
                  }
                }
                n486 = call "Turn to degrees.vi"("Speed/Direction"=-0.95, "Angle"=w891, "RobotDriveDevRef in"=w874) -> ("RobotDriveDevRef out"=w873:T6)  [unwired: 8 in]
                n487 = call-poly <vilib>:"NT Write Value.vi"("Numeric"=3.0, "Name"="Template") -> ()  [unwired: 9 in, 1 out]
                n488 = disable-structure shown="Enabled" {
                  disable-tunnel: w873 -> [w926 w931]
                  disable-tunnel: [w925 w930] -> w898
                  frame Disabled {
                    n489 = call "Forward For inch.vi"("Angle robot facing"=-90.0, "Speed"=-0.6, "Distance"=72.0, "RobotDriveDevRef in"=w926) -> ("RobotDriveDevRef out"=w925:T6)  [unwired: 7 in]
                  }
                  frame Enabled {
                    n490 = disable-structure shown="Disabled" {
                      disable-tunnel: w931 -> [w935 _]
                      frame Disabled {
                        n491 = call "Set Arm Position.vi"("RobotDriveDevRef 2"=w935, "Speed"=0.8, "Setpoint"=550.0) -> ()  [unwired: 8 in, 1 out]
                      }
                      frame Enabled {
                      }
                    }
                    n492 = for {
                      N: 20 -> [_]
                      tunnel: w931 -> [w939]
                      tunnel: [w938] -> w930
                      n493 = call "Drive Straight Arcade.vi"("Angle robot facing"=-80.0) -> ("Arcade drive x"=w936:dbl)  [unwired: 10 in]
                      n494 = Wait (ms)(milliseconds to wait=u32 50) -> ()  [unwired: 1 out]
                      n495 = call-poly <vilib>:"WPI_RobotDriveArcadeDrive.vi"("Y axis value"=-0.55, "X axis value"=w936, "RobotDriveDevRef"=w939) -> ("RobotDriveDevRef"=w938:T6)  [unwired: 6 in, 2 out]
                    }
                  }
                }
                n496 = call "Turn to degrees.vi"("Speed/Direction"=0.7, "Angle"=-65.0, "RobotDriveDevRef in"=w898) -> ("RobotDriveDevRef out"=w890:T6)  [unwired: 8 in]
                n497 = disable-structure shown="Enabled" {
                  disable-tunnel: w890 -> [w944 _]
                  frame Disabled {
                    n498 = call "Set Arm Position.vi"("RobotDriveDevRef 2"=w944, "Speed"=0.9, "Setpoint"=620.0) -> ()  [unwired: 8 in, 1 out]
                  }
                  frame Enabled {
                  }
                }
                n499 = call <vilib>:"WPI_MotorControlRefNum Registry Get.vi"("refnum name"="intakeWheels") -> ("MotorControlDevRef"=w907:T7)  [unwired: 9 in, 1 out]
                n500 = for {
                  N: 20 -> [_]
                  tunnel: w907 -> [w952]
                  tunnel: w896 -> [_]
                  tunnel: w873 -> [_]
                  n501 = Wait (ms)(milliseconds to wait=u32 50) -> ()  [unwired: 1 out]
                  n502 = call <vilib>:"WPI_MotorControlSetOutput.vi"("Output"=-1.0, "MotorControlDevRef"=w952) -> ()  [unwired: 7 in, 3 out]
                }
              }
              frame 2 {
                (unwired) 140.0 ("Camera Angle Vertical")
                (unwired) 145.0 ("Camera Angle")
                w987 = -60.0 ("Angle")
                n503 = call "Set Arm Position.vi"("RobotDriveDevRef 2"=w978, "Setpoint"=350.0) -> ()  [unwired: 9 in, 1 out]
                n504 = call "Turn to degrees.vi"("Speed/Direction"=-0.6, "Angle"=w987, "RobotDriveDevRef in"=w978) -> ("RobotDriveDevRef out"=w991:T6)  [unwired: 8 in]
                n505 = call "Forward For inch.vi"("Angle robot facing"=w987, "Speed"=-0.6, "Distance"=56.0, "RobotDriveDevRef in"=w991) -> ("RobotDriveDevRef out"=w986:T6)  [unwired: 7 in]
                n506 = call "Turn to degrees.vi"("Speed/Direction"=0.6, "Angle"=0.0, "RobotDriveDevRef in"=w986) -> ("RobotDriveDevRef out"=w980:T6)  [unwired: 8 in]
                n507 = call "Set Arm Position.vi"("RobotDriveDevRef 2"=w980, "Speed"=0.8, "Setpoint"=550.0) -> ()  [unwired: 8 in, 1 out]
                n508 = call "Auto Aim.vi"("Turning Angle"=40.0, "RobotDriveDevRef in"=w980, "Angle robot facing"=0.0, "Target Boundries"=cluster{"Upper":dbl, "Lower":dbl} {"Upper"=85.0, "Lower"=78.0}) -> ()  [unwired: 8 in]
              }
              frame 3 {
                w1003 = 80.0 ("Angle")
                # "NEXT TIME MAKE SUBVI FOR THESE SHARED ACTIONS"
                # "may be too much"
                # "Turn and align as if coming out\nof defense 5"
                # "Defense position 3"
                # "disabled case for driving to wall\n at an angle"
                # "Raise arm so it doesn't\ndrag on ground"
                # "This ensures that the intake wheels spit out the boulder with one second left in auto, no matter if the other\nactions (the last turning part is our real concern) finish."
                # "Lower arm"
                # "Shoot"
                n509 = call "Turn to degrees.vi"("Speed/Direction"=0.75, "Angle"=w1003, "RobotDriveDevRef in"=w992) -> ("RobotDriveDevRef out"=w1009:T6)  [unwired: 8 in]
                n510 = call "Forward For inch.vi"("Angle robot facing"=w1003, "Speed"=-0.75, "Distance"=102.0, "RobotDriveDevRef in"=w1009) -> ("RobotDriveDevRef out"=w1008:T6)  [unwired: 7 in]
                n511 = call <vilib>:"WPI_AccelerometerRefNum Registry Get.vi"("refnum name"="accel") -> ("AccelerometerDevRef"=w1029:T14)  [unwired: 9 in, 1 out]
                n512 = while {
                  tunnel: w993 -> [w1042]
                  tunnel: [w1041] -> w1016
                  stop <- w1041 stop-if-true
                  n513 = call "Timeout.vi"("Start Time In"=w1042, "Time Limit"=u32 14000) -> ("Timeout"=w1041:bool)  [unwired: 8 in, 1 out]
                  n514 = Wait (ms)(milliseconds to wait=u32 300) -> ()  [unwired: 1 out]
                }
                n515 = Tick Count (ms)() -> (millisecond timer value=w1022:u32)
                n516 = call "Turn to degrees.vi"("Speed/Direction"=-0.75, "Angle"=0.0, "RobotDriveDevRef in"=w1008) -> ("RobotDriveDevRef out"=w1007:T6)  [unwired: 8 in]
                n517 = while {
                  tunnel: w1029 -> [w1085]
                  tunnel: w1007 -> [w1077]
                  tunnel: [w1076] -> w1019
                  tunnel: [w1075] -> _
                  tunnel: w1022 -> [w1072]
                  stop <- w1074 stop-if-true
                  n518 = disable-structure shown="Enabled" {
                    disable-tunnel: [w1088 0.0 ("X axis value")] -> w1070
                    disable-tunnel: [u32 10000 ("Time Limit") u32 10000 ("Time Limit")] -> w1069
                    frame Enabled {
                      n519 = call "Drive Straight Arcade.vi"("Angle robot facing"=3.0) -> ("Arcade drive x"=w1088:dbl)  [unwired: 10 in]
                    }
                    frame Disabled {
                    }
                  }
                  n520 = call <vilib>:"WPI_AccelerometerGetAcceleration.vi"("AccelerometerDevRef"=w1085) -> ("Accelerations"=w1084:T20, "AccelerometerDevRef"=w1075:T14)  [unwired: 8 in, 1 out]
                  n521 = call "Timeout.vi"("Start Time In"=w1072, "Time Limit"=w1069) -> ("Timeout"=w1071:bool)  [unwired: 8 in, 1 out]
                  n522 = Unbundle By Name(w1084) -> ("Y-Axis"=w1080:dbl)
                  n523 = In Range and Coerce(upper limit=0.8, x=w1080, lower limit=-0.8) -> (In Range?=w1081:bool)  [unwired: 1 out]
                  n524 = Not(x=w1081) -> (.not. x?=w1073:bool)
                  n525 = call-poly <vilib>:"WPI_RobotDriveArcadeDrive.vi"("Y axis value"=-0.65, "X axis value"=w1070, "RobotDriveDevRef"=w1077) -> ("RobotDriveDevRef"=w1076:T6)  [unwired: 6 in, 2 out]
                  n526 = Or(x=w1073, y=w1071) -> (x .or. y?=w1074:bool)
                  n527 = Wait (ms)(milliseconds to wait=u32 20) -> ()  [unwired: 1 out]
                }
                n528 = disable-structure shown="Disabled" {
                  frame Disabled {
                    n529 = call "Turn And Shoot.vi"("Turning Angle"=-95.0) -> ()  [unwired: 11 in]
                  }
                  frame Enabled {
                  }
                }
                n530 = for {
                  N: 1 -> [_]
                  tunnel: [w1061] -> w1018
                  tunnel: w1019 -> [w1061]
                  n531 = Wait (ms)(milliseconds to wait=u32 350) -> ()  [unwired: 1 out]
                }
                n532 = call <vilib>:"WPI_RobotDriveRefNum Registry Get.vi"("refnum name"="intakeDevice") -> ("RobotDriveDevRef"=w999:T6)  [unwired: 9 in, 1 out]
                n533 = call <vilib>:"WPI_SwitchRefNum Registry Get.vi"("refnum name"="mechanismSwitch") -> ("SwitchDevRef"=w996:T12)  [unwired: 9 in, 1 out]
                n534 = call "Forward For inch.vi"("Angle robot facing"=0.0, "Speed"=0.6, "Distance"=-6.0, "RobotDriveDevRef in"=w1018) -> ("RobotDriveDevRef out"=w995:T6)  [unwired: 7 in]
                n535 = for {
                  N: 175 -> [_]
                  tunnel: w999 -> [w1035]
                  tunnel: [w1033] -> _
                  tunnel: w996 -> [w1031]
                  tunnel: w995 -> [_]
                  stop <- w1032 stop-if-true
                  n536 = call <vilib>:"WPI_SwitchGetLimitValue.vi"("SwitchDevRef"=w1031) -> ("Switch Pressed"=w1032:bool)  [unwired: 8 in, 2 out]
                  n537 = call-poly <vilib>:"WPI_RobotDriveArcadeDrive.vi"("Y axis value"=-0.6, "X axis value"=0.0, "RobotDriveDevRef"=w1035) -> ("RobotDriveDevRef"=w1033:T6)  [unwired: 6 in, 2 out]
                  n538 = Wait (ms)(milliseconds to wait=u32 20) -> ()  [unwired: 1 out]
                }
                n539 = disable-structure shown="Enabled" {
                  disable-tunnel: [-100.0 ("Angle") -70.0 ("Angle")] -> w1011
                  frame Disabled {
                  }
                  frame Enabled {
                  }
                }
                n540 = call "Turn to degrees.vi"("Speed/Direction"=-0.9, "Angle"=w1011, "RobotDriveDevRef in"=w995) -> ("RobotDriveDevRef out"=w994:T6)  [unwired: 8 in]
                n541 = call-poly <vilib>:"NT Write Value.vi"("Numeric"=3.0, "Name"="Template") -> ()  [unwired: 9 in, 1 out]
                n542 = disable-structure shown="Enabled" {
                  disable-tunnel: w994 -> [w1045 w1050]
                  disable-tunnel: [w1044 w1049] -> w1017
                  frame Disabled {
                    n543 = call "Forward For inch.vi"("Angle robot facing"=-90.0, "Speed"=-0.6, "Distance"=72.0, "RobotDriveDevRef in"=w1045) -> ("RobotDriveDevRef out"=w1044:T6)  [unwired: 7 in]
                  }
                  frame Enabled {
                    n544 = disable-structure shown="Disabled" {
                      disable-tunnel: w1050 -> [w1054 _]
                      frame Disabled {
                        n545 = call "Set Arm Position.vi"("RobotDriveDevRef 2"=w1054, "Speed"=0.8, "Setpoint"=550.0) -> ()  [unwired: 8 in, 1 out]
                      }
                      frame Enabled {
                      }
                    }
                    n546 = for {
                      N: 20 -> [_]
                      tunnel: w1050 -> [w1058]
                      tunnel: [w1057] -> w1049
                      n547 = call "Drive Straight Arcade.vi"("Angle robot facing"=-80.0) -> ("Arcade drive x"=w1055:dbl)  [unwired: 10 in]
                      n548 = Wait (ms)(milliseconds to wait=u32 50) -> ()  [unwired: 1 out]
                      n549 = call-poly <vilib>:"WPI_RobotDriveArcadeDrive.vi"("Y axis value"=-0.55, "X axis value"=w1055, "RobotDriveDevRef"=w1058) -> ("RobotDriveDevRef"=w1057:T6)  [unwired: 6 in, 2 out]
                    }
                  }
                }
                n550 = call "Turn to degrees.vi"("Speed/Direction"=0.7, "Angle"=-65.0, "RobotDriveDevRef in"=w1017) -> ("RobotDriveDevRef out"=w1010:T6)  [unwired: 8 in]
                n551 = disable-structure shown="Enabled" {
                  disable-tunnel: w1010 -> [w1063 _]
                  frame Disabled {
                    n552 = call "Set Arm Position.vi"("RobotDriveDevRef 2"=w1063, "Speed"=0.9, "Setpoint"=620.0) -> ()  [unwired: 8 in, 1 out]
                  }
                  frame Enabled {
                  }
                }
                n553 = call <vilib>:"WPI_MotorControlRefNum Registry Get.vi"("refnum name"="intakeWheels") -> ("MotorControlDevRef"=w1026:T7)  [unwired: 9 in, 1 out]
                n554 = for {
                  N: 20 -> [_]
                  tunnel: w1026 -> [w1068]
                  tunnel: w1016 -> [_]
                  tunnel: w994 -> [_]
                  n555 = Wait (ms)(milliseconds to wait=u32 50) -> ()  [unwired: 1 out]
                  n556 = call <vilib>:"WPI_MotorControlSetOutput.vi"("Output"=-1.0, "MotorControlDevRef"=w1068) -> ()  [unwired: 7 in, 3 out]
                }
              }
            }
            n557 = call-poly <vilib>:"NT Write Value.vi"("Numeric"=w665, "Name"="Template") -> ()  [unwired: 9 in, 1 out]
          }
        }
        n558 = disable-structure shown="Disabled" {
          frame Disabled {
            # "This slowly pulls the ball in so it doesn't fall out"
            n559 = while {
              stop <- w243 stop-if-true
              n560 = Wait (ms)(milliseconds to wait=u32 50) -> ()  [unwired: 1 out]
              n561 = local read "Stop Wheel Loop"() -> (w243:bool)
              n562 = call <vilib>:"WPI_MotorControlRefNum Registry Get.vi"("refnum name"="intakeWheels") -> ("MotorControlDevRef"=w245:T7)  [unwired: 9 in, 1 out]
              n563 = call <vilib>:"WPI_MotorControlSetOutput.vi"("Output"=0.4, "MotorControlDevRef"=w245) -> ()  [unwired: 7 in, 3 out]
            }
          }
          frame Enabled {
          }
        }
        "Stop Wheel Loop" <- FALSE
      }
      frame 2 {
        # "Shoot here"
        n564 = call <vilib>:"WPI_RobotDriveRefNum Registry Get.vi"("refnum name"="Drive 1") -> ("RobotDriveDevRef"=w1102:T6)  [unwired: 9 in, 1 out]
        n565 = call "Set Arm Position.vi"("RobotDriveDevRef 2"=w1102, "Speed"=0.8, "Setpoint"=550.0) -> ()  [unwired: 8 in, 1 out]
        n566 = call "Forward For inch.vi"("Angle robot facing"=0.0, "Speed"=-0.65, "Distance"=90.0, "RobotDriveDevRef in"=w1102) -> ("RobotDriveDevRef out"=w1093:T6)  [unwired: 7 in]
        n567 = call-poly <vilib>:"NT Write Value.vi"("Numeric"=3.0, "Name"="Template") -> ()  [unwired: 9 in, 1 out]
        n568 = call <vilib>:"WPI_MotorControlRefNum Registry Get.vi"("refnum name"="intakeWheels") -> ("error out"=w1094:errorcluster, "MotorControlDevRef"=w1095:T7)  [unwired: 9 in]
        n569 = for {
          N: 20 -> [_]
          tunnel: w1094 -> [w1110]
          tunnel: w1095 -> [w1109]
          tunnel: w1093 -> [_]
          n570 = Wait (ms)(milliseconds to wait=u32 50) -> ()  [unwired: 1 out]
          n571 = call <vilib>:"WPI_MotorControlSetOutput.vi"("error in (no error)"=w1110, "Output"=-1.0, "MotorControlDevRef"=w1109) -> ()  [unwired: 6 in, 3 out]
        }
      }
    }
  }
